vi "4ChNCS_BIOPAC_dyspnea.vi"() -> ()   [LabVIEW 2016]
uses:
  <instrlib>/niUSRP/niUSRP Timestamp.ctl
  <vilib>/Utility/miscctls.llb/LVDateTimeRec.ctl
  <vilib>/Analysis/3filter.llb/Filter Passband Type.ctl
  <vilib>/sound2/lvsound2.llb/Sampling Mode.ctl
  <instrlib>/niUSRP/niUSRP Configure Time Start Trigger.vi
  <vilib>/Platform/browser.llb/Open URL in Default Browser (string).vi
  <instrlib>/niUSRP/niUSRP Write Tx Data (2D CDB).vi
  <instrlib>/niUSRP/niUSRP Fetch Rx Data (2D CDB).vi
  <vilib>/Analysis/3filter.llb/Butterworth Filter (DBL).vi
  <vilib>/Analysis/3filter.llb/Butterworth Filter (CDB).vi
  <vilib>/sound2/lvsound2.llb/Sound File Info (path).vi
  <vilib>/sound2/lvsound2.llb/Sound File Read Open.vi
  <vilib>/sound2/lvsound2.llb/Sound File Read (DBL).vi
  <vilib>/sound2/lvsound2.llb/Sound Output Write (DBL).vi
  <vilib>/measure/NI_MABase.lvlib
  <vilib>/Analysis/NI_AALBase.lvlib
  Program Files (x86)/BIOPAC Systems, Inc/BIOPAC Hardware API 2.2 Education/x64/mpdev.dll
panel:
  in  "Mute":bool
  out "Play Sound":bool=TRUE
  in  "bottom filter":T1
  in  "top filter":T1=enum."Bandpass"
  out "Acq Started":bool
  out "# BIO View Q":i32
  out "# BIO Buffer":i32
  out "Boolean":bool=TRUE
  out "Disconnecting":bool
  out "Stopping":bool
  out "Connecting":bool
  out "Disconnected":bool
  in  "Show BIO":bool
  out "# BIOViewQ2":i32
  out "Array 1 View":dbl[](graph)
  out "Array 2 View":dbl[](graph)
  out "Array 3 View":dbl[](graph)
  out "Array 4 View":dbl[](graph)
  out "View Array Size":i32
  out "# Elements in Array":i32
  out "ACQ -# Elements":i32
  out "Receive Success":bool
  out "# ACQ cycles":i32
  out "Bytes Read":i32
  out "Bytes To Read":i32
  out "Receive Total Size":dbl format="%#_13g"
  out "Receiving":bool
  in  "Start Acquisition":bool
  in  "Disconnect":bool
  out "ACQ ms":dbl=250.0 format="%#_13g"
  in  "Stop Acquisition":bool
  out "Connected":bool
  in  "Sample Rate":dbl=1.0 caption="ms/sample" min=0.0
  in  "Analog Channels":i32[](array[numeric])=[1, 1, 1, 1]
  out "# Channels":dbl format="%#_13g"
  out "BIO Connect":i32
  in  "BIO Connect":bool=TRUE
  in  "OpenHTML":bool=TRUE
  in  "Abd (cm)":string="0"
  in  "Thorax (cm)":string="0"
  in  "Comments":string
  in  "Weight (lbs)":string="0"
  in  "Age (yrs)":string="0"
  in  "Sex":string(combo)="Female"
  in  "Height (cm)":string="0"
  in  "Case #":string="0"
  out "Start Time":T2
  out "Total Routine Time":dbl(slide) scale=0.0..300.0
  out "Elapsed Time":dbl caption="Elapsed Time (s)"
  out "Next Instruction":string
  out "Current Instruction":string
  in  "Routine Selection":T3(ring)
  out "Current Routine":string
  out "Tx3Rx4":dbl[](graph)
  out "Tx4Rx4":dbl[](graph)
  out "Tx4Rx3":dbl[](graph)
  out "Tx3Rx3":dbl[](graph)
  out "ChAmp":dbl[][](array[numeric])=[[1.7262327066457893e-05, 1.899698926539768e-05, 2.131979680782845e-05, 2.7507513862708948e-05, 3.236234947998919e-05, 3.384280863448985e-05, 3.3113712649913256e-05, 2.8744318806479064e-05, 2.4117959107532184e-05, 2.0714217164135817e-05, 1.7964639969242282e-05, 1.4127881869429752e-05, 1.5692535768228094e-05, 2.4152619914305532e-05, 2.8339686382715385e-05, 2.606906286720416e-05, 2.1755918570529384e-05, 2.0929028564145826e-05, 2.2419410493859248e-05, 2.1786896096171967e-05, 1.7145005999174206e-05, 1.5886785364638103e-05, 1.995380091360238e-05, 1.96084446445408e-05, 1.3881312052638574e-05, 5.368463432831762e-06, 7.886976522489036e-06, 1.718108126568357e-05, 1.984430714817916e-05, 1.8874058751572535e-05, 1.7869312672433515e-05, 1.7356735499504872e-05, 2.065235332503479e-05, 2.1951680154988656e-05, 2.0363547237431346e-05, 2.1229264430323524e-05, 2.188656276617781e-05, 2.1477411495382004e-05, 1.913194947952161e-05, 1.374906879007994e-05, 1.084407557924396e-05, 1.0538448835067238e-05, 1.3462486513328936e-05, 1.979383250422823e-05, 2.381539261154395e-05, 2.2167223174073578e-05, 1.7644503717147575e-05, 1.870536234643517e-05, 2.2751950524913166e-05, 2.340432192813861e-05, 2.2468849270761083e-05, 2.4188550691353842e-05, 2.7519058552290856e-05, 3.1102581077866726e-05, 3.580393911829494e-05, 3.78912649503874e-05, 3.327873597801261e-05, 2.4510981949940783e-05, 1.8465065354817837e-05, 1.7132224969133005e-05, 1.7642310138371268e-05, 1.88142956741822e-05, 1.560032046277488e-05, 9.753217862235494e-06, 1.2015090850038981e-05, 1.776834560720681e-05, 2.4803861691952522e-05, 2.8043624192078222e-05, 2.684382525540612e-05, 2.3530222840588965e-05, 2.0528849124310057e-05, 1.9668374613316667e-05, 1.9146637114645684e-05, 1.5474488036915515e-05, 1.739488550213199e-05, 2.5095299380068926e-05, 3.2858145215540916e-05, 3.439509649081835e-05, 2.6143868318774837e-05, 1.7977385637690134e-05, 1.6384181575586158e-05, 1.4888284293264162e-05, 1.1597491470576354e-05, 1.1445555578759772e-05, 1.4980688444081562e-05, 1.909173519498907e-05, 1.9461150455264684e-05, 1.845876729070065e-05, 1.8005010185132642e-05, 1.9028924898462435e-05, 1.7575955788217445e-05, 1.4184298105937452e-05, 9.414371560237339e-06, 5.4356042784590255e-06, 8.10928562517548e-06, 9.28876849225871e-06, 8.695785214389758e-06, 1.2695777397634576e-05, 1.6809431598631123e-05, 2.1908643727461497e-05], [0.39904903865563796, 0.39903176051530775, 0.39902405260596024, 0.3990221650023599, 0.3990182934858042, 0.39901299641778676, 0.39900459263010085, 0.39899398548309095, 0.3989851312683333, 0.3989817758172843, 0.39898441600096285, 0.3989920701551657, 0.3989957319087615, 0.3989970252526829, 0.3990014639144786, 0.3990082495650084, 0.39901677157837184, 0.39902202434845035, 0.3990170521098724, 0.3990061914814684, 0.39899957115083645, 0.39900163440594105, 0.39901134932465093, 0.3990245430143365, 0.3990299364956871, 0.3990206423396574, 0.39901294696264844, 0.399015237964853, 0.3990195320664335, 0.3990239908891069, 0.39902678858482366, 0.3990303142377581, 0.3990363654196349, 0.39903798034344395, 0.39903568308022536, 0.3990295778239386, 0.3990213145612541, 0.3990115641317417, 0.3990031911721688, 0.3990044335692754, 0.3990142055365442, 0.3990231880559529, 0.3990294810791408, 0.39903152543597487, 0.3990303417237137, 0.39902587131491124, 0.39902317862698444, 0.3990231908517323, 0.3990187535042287, 0.39901147460102687, 0.39900466569609977, 0.399000198693456, 0.398994572076958, 0.39898792975360287, 0.39898351183081265, 0.39898252129559103, 0.3989860199605185, 0.3989908704807006, 0.39899345184972185, 0.39899268675930705, 0.39898929894357515, 0.39898974479144206, 0.3989970434213525, 0.39900457970685, 0.3990084272376425, 0.3990059437407563, 0.39900092658003017, 0.3989998521554356, 0.3989999155043143, 0.39900335732390085, 0.3990086633280822, 0.39901161043288735, 0.3990153435576799, 0.3990232290578827, 0.39902895125044885, 0.3990233171970213, 0.39901091768095076, 0.3989963560226853, 0.3989823146041765, 0.39898013105698543, 0.39899131681473166, 0.3990088743561722, 0.39902163871137375, 0.39902552269435965, 0.3990216751013488, 0.3990108271690995, 0.3989999368161602, 0.39899179748001445, 0.3989869444795569, 0.3989823014007489, 0.3989811018380635, 0.3989866085692465, 0.3989974881575293, 0.399009653455826, 0.39902039237597164, 0.39903113834388676, 0.39903799466445666, 0.39903656085835637, 0.39902912933239515, 0.3990196685727854], [0.5089284260094796, 0.5089413529092005, 0.5089385924023097, 0.5089461735853302, 0.5089333321440155, 0.5089367652503622, 0.5089376331435306, 0.5089306671430541, 0.508949239645895, 0.5089486561361645, 0.5089529378833244, 0.5089419476875585, 0.5089298840108731, 0.5089475772042052, 0.5089441426339854, 0.5089427381450184, 0.5089483329108746, 0.5089280151098653, 0.5089336602793385, 0.5089062019851882, 0.5089074628030626, 0.5088932174425751, 0.5088701289561509, 0.5088760830698362, 0.5088683341509143, 0.5088818393635381, 0.5089000365985035, 0.5088962730652971, 0.5089053012825656, 0.5088919060061875, 0.5088858810710211, 0.5088778714303226, 0.508862396898039, 0.5088799706522465, 0.508890020250467, 0.5089068411749241, 0.508910151200762, 0.5088879724716624, 0.5088963605339264, 0.5088989546591678, 0.5089079531975655, 0.5089307483176185, 0.5089353690581762, 0.5089322510910641, 0.5089226818391756, 0.5089231205950179, 0.5089421889187917, 0.5089302121637822, 0.5089288553338916, 0.5089136387417116, 0.5088923938634197, 0.5088806790242092, 0.5088543127997475, 0.5088388632427274, 0.5088290815518671, 0.5088136498514574, 0.508828716232115, 0.5088373004254244, 0.5088536031198835, 0.5088663652543981, 0.5088663647379902, 0.5088663839922184, 0.5088589552438861, 0.5088642449634635, 0.5088725023266256, 0.5088718014416865, 0.5088674063260687, 0.5088515437004615, 0.5088682831786894, 0.5088713788197812, 0.5088809924897628, 0.508878513506942, 0.5088771181893693, 0.5088848435184512, 0.5088770842370816, 0.5088914766511436, 0.5089003523667647, 0.5089066301516674, 0.5089314320882471, 0.5089402101447223, 0.508962553406896, 0.5089753861787446, 0.5089593307295952, 0.5089478542324088, 0.5089278310589712, 0.5089248500720587, 0.5089163513653545, 0.5089005689237424, 0.5089083211616405, 0.5088993300683022, 0.5088927412237987, 0.5088830866377116, 0.5088718481995638, 0.5088897909905771, 0.5088809733102648, 0.5088790935282286, 0.5088680814653207, 0.5088523600270333, 0.5088613943195607, 0.5088543176402154], [2.0662941946213977e-05, 2.282608405319783e-05, 2.237600508813514e-05, 2.2542693256186783e-05, 2.041826329305299e-05, 1.6288400811782785e-05, 1.0891495139698275e-05, 1.4190599881567273e-05, 1.8742691366266016e-05, 1.8736119036749436e-05, 1.741774537028846e-05, 1.5658954058158222e-05, 1.5904856683822096e-05, 1.6871005066910787e-05, 1.5599249074465836e-05, 1.3520520470394872e-05, 1.3927163947888679e-05, 1.5334805249818678e-05, 1.4564830067379515e-05, 9.817520346860189e-06, 1.3098820613974226e-05, 1.929550220456421e-05, 2.3072255815616586e-05, 2.4321951176986116e-05, 2.3250917563816834e-05, 2.1644284217119052e-05, 1.7041306350033735e-05, 1.0688883027066213e-05, 9.28433634468159e-06, 1.1420718289762068e-05, 1.7056250213804775e-05, 1.9836991189555113e-05, 1.746716828521344e-05, 1.2441527630540996e-05, 8.566795426917848e-06, 9.815076354382859e-06, 1.0229272880058857e-05, 9.936691802926115e-06, 1.536494187514889e-05, 2.3346259934086635e-05, 2.7477587888222747e-05, 2.882421007601368e-05, 2.763067836551142e-05, 2.1577345489474273e-05, 1.3485424327083916e-05, 9.52579824483287e-06, 1.3113651673496717e-05, 1.5276095683726537e-05, 1.6308973250379756e-05, 1.8045078515596545e-05, 1.7849042225306495e-05, 1.2607829522468473e-05, 7.109107971268437e-06, 6.6038815895810515e-06, 6.924972052119899e-06, 4.965235247536195e-06, 5.757305113334596e-06, 9.21497446069365e-06, 9.781248515919794e-06, 1.0683021318304504e-05, 1.196938592791573e-05, 1.159802409297526e-05, 1.012272777630437e-05, 9.65935822948268e-06, 1.4116839432017005e-05, 1.847684147148342e-05, 1.6783927528588872e-05, 1.0863513026975652e-05, 7.650914818223192e-06, 9.456183557358687e-06, 1.0426180609097815e-05, 8.567604650724215e-06, 8.546559610017728e-06, 1.2946532793024891e-05, 1.7245567743458815e-05, 2.0097444147186203e-05, 2.0459407417437442e-05, 1.9957232554286306e-05, 1.996659645997603e-05, 1.7332136966233293e-05, 1.5115608112097958e-05, 1.762095864401886e-05, 1.992020410454883e-05, 2.0585166404108466e-05, 2.212056735942569e-05, 2.2957279986002272e-05, 2.3103396847026532e-05, 2.320807116373638e-05, 2.0818984342366494e-05, 1.789850158592137e-05, 1.64936985167028e-05, 1.4204813599995013e-05, 1.2878752736428332e-05, 1.4757379916553103e-05, 1.713867099725903e-05, 1.6105166890214558e-05, 1.20593443919334e-05, 1.2171370167939264e-05, 1.2336933066341984e-05, 1.1620987924410626e-05]]
  out "Output":bool=TRUE
  out "Ch4 Amplitude":dbl step=0.05 format="%#.6g"
  out "Ch3 Amplitude":dbl=0.25 step=0.05 format="%#.6g"
  out "Ch2 Amplitude":dbl=0.6 step=0.05 format="%#.6g"
  out "Ch1 Amplitude":dbl step=0.05 format="%#.6g"
  out "Tx1Rx2":dbl[](graph)
  out "Tx2Rx2":dbl[](graph)
  out "Tx2Rx1":dbl[](graph)
  out "Dis Sampling Rate":dbl=1000.0 format="%#_6p"
  in  "DownSamplingRatio 2":i32=10
  out "Sampling Rate":dbl=10000.0 format="%#_6p"
  out "Flush":bool
  out "8 Ch Heart":dbl[][](array[numeric])
  out "NCS Save Loops":i32=56132
  out "Save":bool
  out "# NCS Buffer":i32
  out "Buffer":bool
  in  "fl Bottom":dbl=10.0 format="%0.4f"
  in  "fh Bottom":dbl=20.0 format="%0.2f"
  in  "DownSamplingRatio1":i32=100
  in  "fl Top":dbl=4.0 format="%0.4f"
  in  "fh Top":dbl=20.0 format="%0.2f"
  out "# elements in view queue":i32
  out "Tx1Rx1":dbl[](graph)
  out "DownSamplingRatio":i32=100
  out "BW/2":dbl=1000.0
  out "# IQ queue Ch 2":i32
  out "# IQ queue Ch 1":i32
  in  "Dis2":bool=TRUE
  in  "Dis1":bool=TRUE
  out "IQ Graph 2":dbl[][](graph)
  out "IQ Graph":dbl[][](graph)
  out "Tx2 Waveform":cdb[][](array[numeric])
  out "Tx1 Waveform":cdb[][](array[numeric])
  in  "Ch3&4 carrier frequency [Hz] 2":dbl=1830000000.0 format="%#_6p"
  in  "Ch1&2 carrier frequency [Hz]":dbl=900000000.0 format="%#_6p"
  in  "Rx2 Gain 2":dbl=5.0 format="%#_6f"
  in  "Tx2 Gain 2":dbl=5.0 format="%#_6f"
  in  "Rx1 Gain 2":dbl=20.0 format="%#_6f"
  in  "Tx1 Gain 2":dbl=20.0 format="%#_6f"
  out "error out 2":errorcluster
  in  "Start Trigger Time 2":T4={"whole seconds"=1, "fractional seconds"=0.0}
  in  "Channel 4 Tone Amplitude":dbl=0.5 step=0.05 format="%#.6g"
  in  "Channel 4 Tone Frequency":dbl=430000.0 format="%#_6p"
  in  "Channel 3 Tone Amplitude":dbl=0.5 step=0.05 format="%#.6g"
  in  "Channel 3 Tone Frequency":dbl=473000.0 format="%#_6p"
  out "Tx2 Waveform Graph":waveform(dbl)[](graph)=[{"t0"=timestamp(0.45999999999999996 s since 1904-01-01), "dt"=1e-06, "Y"=array[10000 elements]}, {"t0"=timestamp(0.45999999999999996 s since 1904-01-01), "dt"=1e-06, "Y"=array[10000 elements]}, {"t0"=timestamp(0.45999999999999996 s since 1904-01-01), "dt"=1e-06, "Y"=array[10000 elements]}, {"t0"=timestamp(0.45999999999999996 s since 1904-01-01), "dt"=1e-06, "Y"=array[10000 elements]}]
  in  "Waveform Size 2":dbl=10000.0
  in  "Stop 2":bool
  in  "Device Name 2":refnum<k15>="MyB210_2"
  in  "Tx2 Gain 1":dbl=5.0 format="%#_6f"
  in  "Tx IQ Rate 2":dbl=1000000.0 format="%#_6p"
  in  "Rx2 Gain 1":dbl=5.0 format="%#_6f"
  in  "Rx IQ Rate 2":dbl=1000000.0 format="%#_6p"
  out "error out 1":errorcluster
  in  "Start Trigger Time":T4={"whole seconds"=1, "fractional seconds"=0.0}
  in  "Stop":bool
  in  "Channel 2 Tone Amplitude":dbl=0.5 step=0.05 format="%#.6g"
  in  "Channel 2 Tone Frequency":dbl=440000.0 format="%#_6p"
  in  "Channel 1 Tone Amplitude":dbl=0.5 step=0.05 format="%#.6g"
  in  "Channel 1 Tone Frequency":dbl=355000.0 format="%#_6p"
  out "Tx1 Waveform Graph":waveform(dbl)[](graph)=[{"t0"=timestamp(0.45999999999999996 s since 1904-01-01), "dt"=1e-06, "Y"=array[10000 elements]}, {"t0"=timestamp(0.45999999999999996 s since 1904-01-01), "dt"=1e-06, "Y"=array[10000 elements]}, {"t0"=timestamp(0.45999999999999996 s since 1904-01-01), "dt"=1e-06, "Y"=array[10000 elements]}, {"t0"=timestamp(0.45999999999999996 s since 1904-01-01), "dt"=1e-06, "Y"=array[10000 elements]}]
  in  "Waveform Size 1":dbl=10000.0
  in  "Device Name":refnum<k15>="MyB210_1"
  in  "Tx1 Gain 1":dbl=20.0 format="%#_6f"
  in  "Tx IQ Rate 1":dbl=1000000.0 format="%#_6p"
  in  "Rx1 Gain 1":dbl=20.0 format="%#_6f"
  in  "Rx IQ Rate 1":dbl=1000000.0 format="%#_6p"
  # "Misc"
  # "Tx Waveform"
  # "IQ waveform"
  # "NCS"
  # "Channel Settings"
  # "Channel 1"
  # "Device Settings"
  # "BIO"
  # "Channel 2"
  # "Filters"
  # "Buffers"
  # "BIOPAC Connection"
  # "Channel 3"
  # "Post Study Survey:"
  # "https://cornell.qualtrics.com/jfe/form/SV_9QryoqkUKquSXD7"
  # "Channel 4"
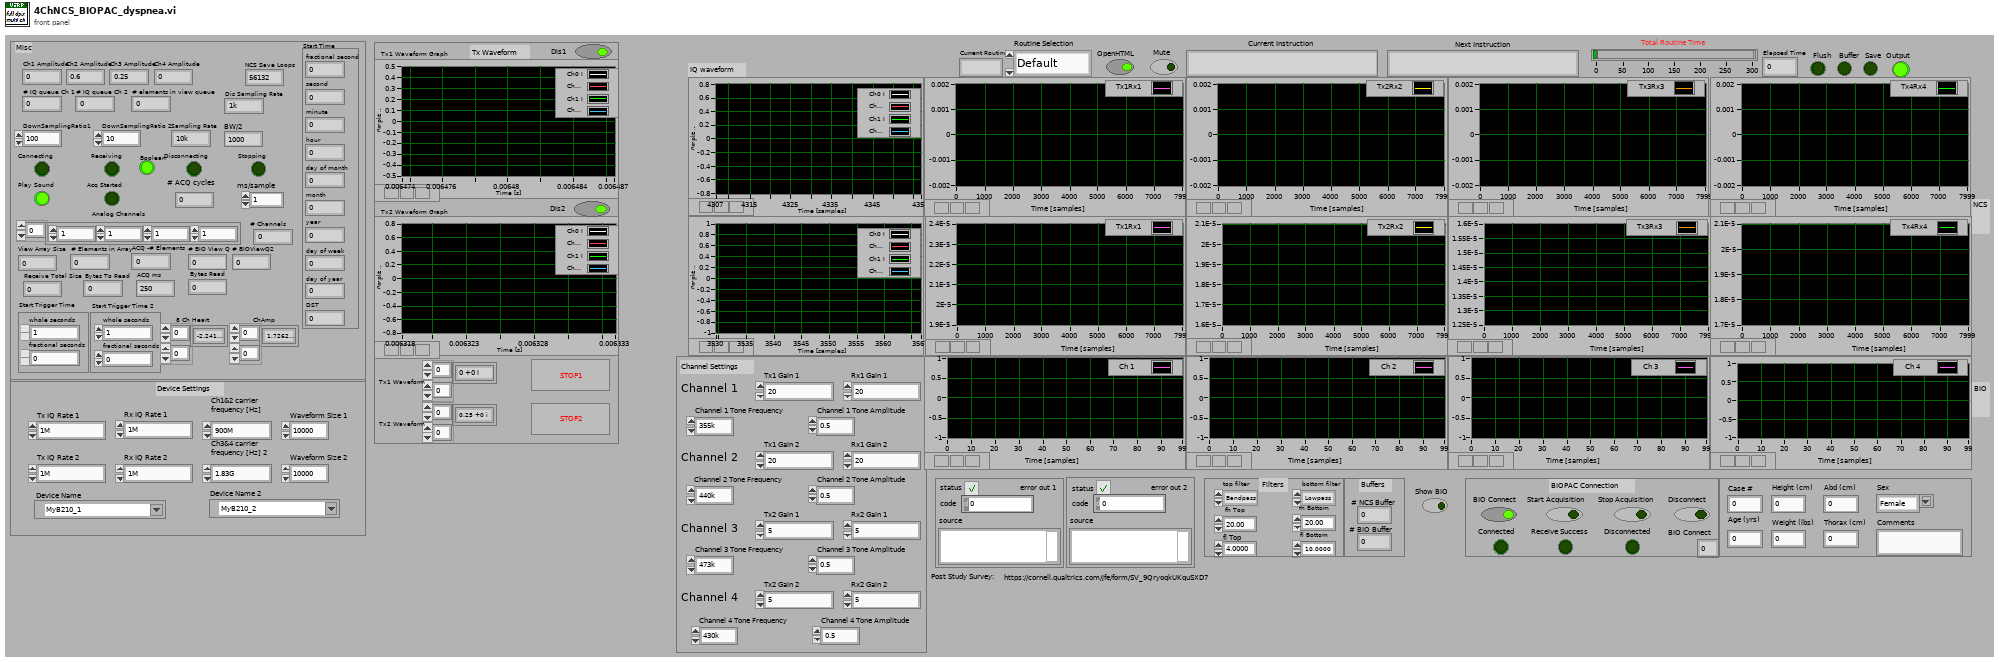
[diagram p1: front panel]
types:
  T1 = typedef "NI_AALBase.lvlib/Filter Passband Type.ctl" = enum32{"Lowpass", "Highpass", "Bandpass", "Bandstop"}
  T2 = typedef "LVDateTimeRec.ctl" = cluster{"fractional second":dbl, "second":i32, "minute":i32, "hour":i32, "day of month":i32, "month":i32, "year":i32, "day of week":i32, "day of year":i32, "DST":i32}
  T3 = enum16{"Default", "Test Run", "Training", "Routine 1", "Routine 2", "Routine 3", "Routine 4", "Routine 5a", "Routine 5b"}
  T4 = typedef "niUSRP Timestamp.ctl" = cluster{"whole seconds":u64, "fractional seconds":dbl}
  T5 = typedef "Sampling Mode.ctl" = i32
  T6 = typedef "Sound Data Format.ctl" = cluster{"sample rate (S/s)":dbl, "number of channels":i32, "bits per sample":i32}
  T7 = typedef "Sound File Refnum.ctl" = refnum<file>
  T8 = typedef "Sound Output Task ID.ctl" = u32
  T9 = enum16{"open", "open or create", "create or replace", "create", "open (read-only)"}
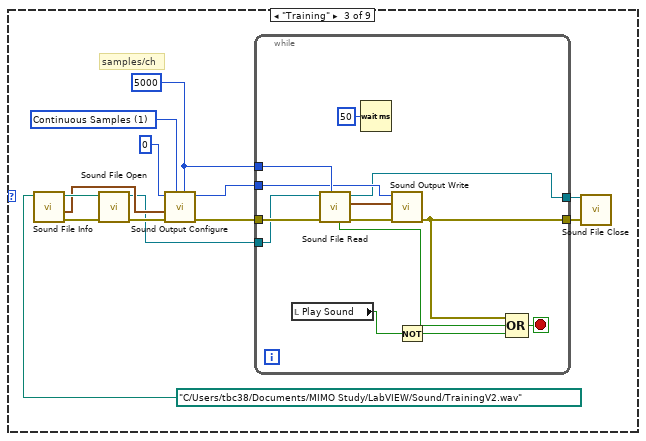
[diagram p5: hidden frame]
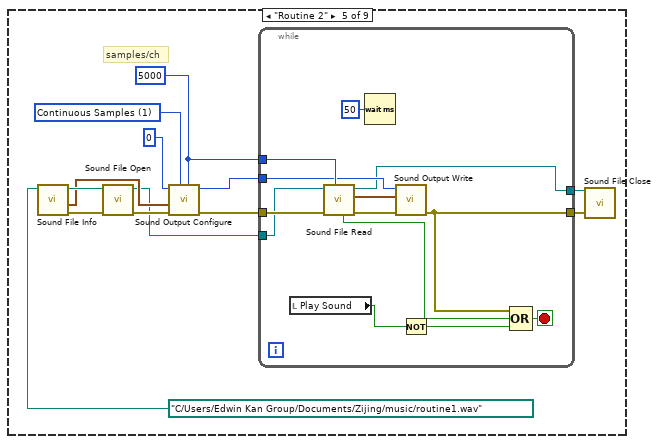
[diagram p7: hidden frame]
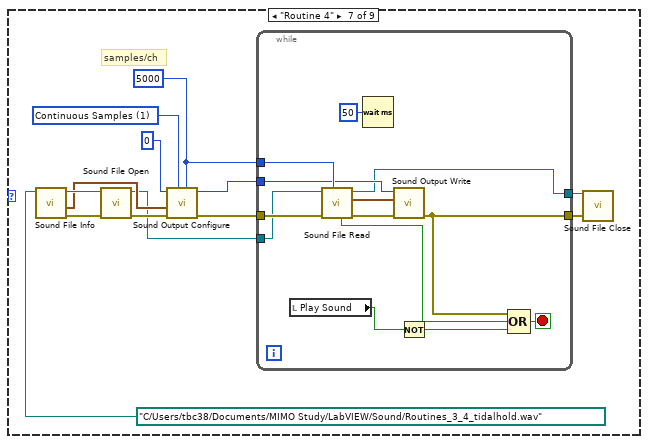
[diagram p8: hidden frame]
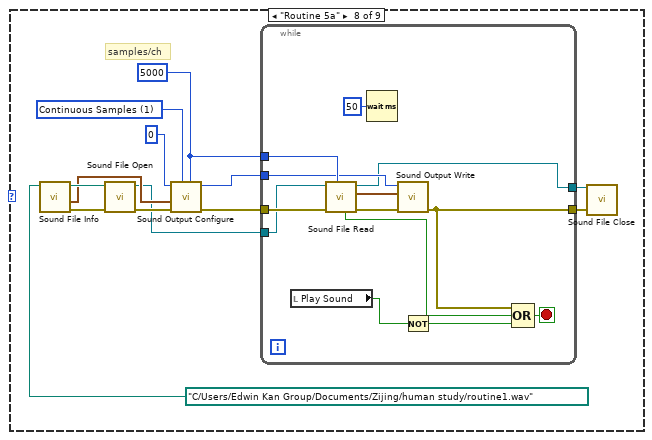
[diagram p9: hidden frame]
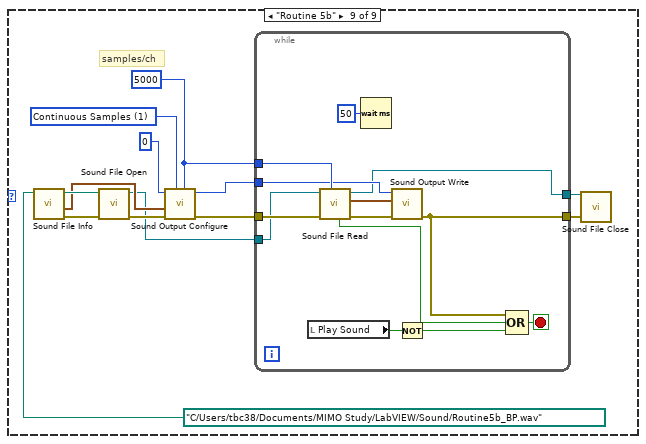
[diagram p10: hidden frame]
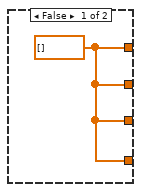
[diagram p11: hidden frame]
diagram:
  w1 = FALSE
  w29 = enum16{"Default"}."Default"
  w26 = 0.0 ("element")
  w27 = 800 ("dimension size")
  w33 = 4 ("dimension size")
  (unwired) 10
  w85 = "RX2"  # Tx active antenna
  w86 = "RX2"  # Tx active antenna
  w142 = 1 items=["Now", "Next Timebase Edge"] ("apply timestamp")
  w114 = "TX1"  # Tx active antenna
  w208 = 1 items=["Now", "Next Timebase Edge"] ("apply timestamp")
  w180 = "TX1"  # Tx active antenna
  # "Sound"
  # "Get it so that it acquires the proper number of cycles for the routine time. Front should be save synchronized"
  # "BIOPAC QUEUE"
  # "Current Sync Method:\nStart Buffering as soon as Acquisition Starts"
  # "Biopac Code. Use the flags to switch between these loops.\nCONNECT- Run to connect to the BIOPAC. Acquisition will not start. 'Connect Success' returns the status of this function.\nSTART ACQUISITION- Run to begin acquiring data from the BIOPAC. SYNCHRONIZATION IS IMPORTANT HERE.\nSTOP ACQUISITION- Run to stop acquiring data. The BIOPAC will disconnect and reconnect to prepare for another acquisition.\nDISCONNECT- Run to disconnect from BIOPAC. This will prohibit connection until the VI is restarted.\nSHOW/VIEWING- Dequeues the elements and displays them."
  # "Routine selection and implementation Loop"
  # "DownSamplingRatio"
  # "Set the attributes \nspecific to channel 1."
  # "Set the attributes \nspecific to channel 0."
  # "Set the attributes \nused by both Rx channels"
  # "Set the attributes \nspecific to Rx channel 1."
  # "Set the attributes \nspecific to Rx channel 0."
  # "Set the attributes \nspecific to channel 1."
  # "Set the attributes \nspecific to channel 0."
  # "Set the attributes \nused by both Rx channels"
  # "Set the attributes \nspecific to Rx channel 1."
  # "Set the attributes \nspecific to Rx channel 0."
  n1 = local write "BIO Connect"(w1) -> ()
  n2 = local write "Start Acquisition"(w1) -> ()
  n3 = local write "Stop Acquisition"(w1) -> ()
  n4 = local write "Disconnect"(w1) -> ()
  n5 = local write "Show BIO"(w1) -> ()
  n6 = local read "Device Name 2"() -> (w150:refnum<k15>)
  n7 = while {
    stop <- FALSE stop-if-true
    n8 = Wait (ms)(milliseconds to wait=50) -> ()  [unwired: 1 out]
    n9 = Not(x="Mute") -> (.not. x?=w224:bool)
    n10 = case shown="True" w224 {
      frame False {
      }
      frame True {
        n11 = local read "Routine Selection"() -> (w227:T3)
        n12 = case shown="\"Routine 3\"" w227 {
          frame "Default", Default {
          }
          frame "Test Run" {
          }
          frame "Training" {
            w231 = 5000
            w234 = T5 1 items=["Finite Samples", "Continuous Samples"] ("sample mode")
            # "samples/ch"
            n13 = call-poly <vilib>:"Sound File Info.vi"("path"=path "C:/Users/tbc38/Documents/MIMO Study/LabVIEW/Sound/TrainingV2.wav") -> ("error out"=w239:errorcluster, "sound format"=w235:T6, "path out"=w240:path)  [unwired: 7 in, 1 out]
            n14 = call-poly <vilib>:"Sound File Open.vi"("error in (no error)"=w239, "path"=w240) -> ("error out"=w238:errorcluster, "sound file refnum"=w230:T7)  [unwired: 8 in]
            n15 = call <vilib>:"Sound Output Configure.vi"("number of samples/ch"=w231, "sample mode"=w234, "error in (no error)"=w238, "sound format"=w235, "device ID"=u32 0) -> ("error out"=w233:errorcluster, "task ID"=w232:T8)  [unwired: 5 in]
            n16 = while {
              tunnel: w233 -> [w251]
              tunnel: w232 -> [w252]
              tunnel: w231 -> [w253]
              tunnel: w230 -> [w250]
              tunnel: [w244] -> w229
              tunnel: [w248] -> w228
              stop <- w242 stop-if-true
              n17 = local read "Play Sound"() -> (w241:bool)
              n18 = call-poly <vilib>:"Sound File Read.vi"("number of samples/ch (-1: all)"=w253, "error in (no error)"=w251, "sound file refnum"=w250) -> ("error out"=w247:errorcluster, "data"=w246:waveform(dbl)[], "sound file refnum out"=w248:T7, "end of file?"=w245:bool)  [unwired: 4 in, 1 out]
              n19 = Wait (ms)(milliseconds to wait=50) -> ()  [unwired: 1 out]
              n20 = call-poly <vilib>:"Sound Output Write.vi"("error in (no error)"=w247, "data"=w246, "task ID"=w252) -> ("error out"=w244:errorcluster)  [unwired: 7 in, 1 out]
              n21 = Not(x=w241) -> (.not. x?=w243:bool)
              n22 = Compound Arithmetic op=OR(w244, w245, w243) -> (w242:bool)
            }
            n23 = call <vilib>:"Sound File Close.vi"("error in (no error)"=w229, "sound file refnum"=w228) -> ()  [unwired: 9 in, 1 out]
          }
          frame "Routine 1" {
          }
          frame "Routine 2" {
            w257 = 5000
            w260 = T5 1 items=["Finite Samples", "Continuous Samples"] ("sample mode")
            # "samples/ch"
            n24 = call-poly <vilib>:"Sound File Info.vi"("path"=path "C:/Users/Edwin Kan Group/Documents/Zijing/music/routine1.wav") -> ("error out"=w265:errorcluster, "sound format"=w261:T6, "path out"=w266:path)  [unwired: 7 in, 1 out]
            n25 = call-poly <vilib>:"Sound File Open.vi"("error in (no error)"=w265, "path"=w266) -> ("error out"=w264:errorcluster, "sound file refnum"=w256:T7)  [unwired: 8 in]
            n26 = call <vilib>:"Sound Output Configure.vi"("number of samples/ch"=w257, "sample mode"=w260, "error in (no error)"=w264, "sound format"=w261, "device ID"=u32 0) -> ("error out"=w259:errorcluster, "task ID"=w258:T8)  [unwired: 5 in]
            n27 = while {
              tunnel: w259 -> [w277]
              tunnel: w258 -> [w278]
              tunnel: w257 -> [w279]
              tunnel: w256 -> [w276]
              tunnel: [w270] -> w255
              tunnel: [w274] -> w254
              stop <- w268 stop-if-true
              n28 = local read "Play Sound"() -> (w267:bool)
              n29 = call-poly <vilib>:"Sound File Read.vi"("number of samples/ch (-1: all)"=w279, "error in (no error)"=w277, "sound file refnum"=w276) -> ("error out"=w273:errorcluster, "data"=w272:waveform(dbl)[], "sound file refnum out"=w274:T7, "end of file?"=w271:bool)  [unwired: 4 in, 1 out]
              n30 = Wait (ms)(milliseconds to wait=50) -> ()  [unwired: 1 out]
              n31 = call-poly <vilib>:"Sound Output Write.vi"("error in (no error)"=w273, "data"=w272, "task ID"=w278) -> ("error out"=w270:errorcluster)  [unwired: 7 in, 1 out]
              n32 = Not(x=w267) -> (.not. x?=w269:bool)
              n33 = Compound Arithmetic op=OR(w270, w271, w269) -> (w268:bool)
            }
            n34 = call <vilib>:"Sound File Close.vi"("error in (no error)"=w255, "sound file refnum"=w254) -> ()  [unwired: 9 in, 1 out]
          }
          frame "Routine 3" {
          }
          frame "Routine 4" {
            w283 = 5000
            w286 = T5 1 items=["Finite Samples", "Continuous Samples"] ("sample mode")
            # "samples/ch"
            n35 = call-poly <vilib>:"Sound File Info.vi"("path"=path "C:/Users/tbc38/Documents/MIMO Study/LabVIEW/Sound/Routines_3_4_tidalhold.wav") -> ("error out"=w291:errorcluster, "sound format"=w287:T6, "path out"=w292:path)  [unwired: 7 in, 1 out]
            n36 = call-poly <vilib>:"Sound File Open.vi"("error in (no error)"=w291, "path"=w292) -> ("error out"=w290:errorcluster, "sound file refnum"=w282:T7)  [unwired: 8 in]
            n37 = call <vilib>:"Sound Output Configure.vi"("number of samples/ch"=w283, "sample mode"=w286, "error in (no error)"=w290, "sound format"=w287, "device ID"=u32 0) -> ("error out"=w285:errorcluster, "task ID"=w284:T8)  [unwired: 5 in]
            n38 = while {
              tunnel: w285 -> [w303]
              tunnel: w284 -> [w304]
              tunnel: w283 -> [w305]
              tunnel: w282 -> [w302]
              tunnel: [w296] -> w281
              tunnel: [w300] -> w280
              stop <- w294 stop-if-true
              n39 = local read "Play Sound"() -> (w293:bool)
              n40 = call-poly <vilib>:"Sound File Read.vi"("number of samples/ch (-1: all)"=w305, "error in (no error)"=w303, "sound file refnum"=w302) -> ("error out"=w299:errorcluster, "data"=w298:waveform(dbl)[], "sound file refnum out"=w300:T7, "end of file?"=w297:bool)  [unwired: 4 in, 1 out]
              n41 = Wait (ms)(milliseconds to wait=50) -> ()  [unwired: 1 out]
              n42 = call-poly <vilib>:"Sound Output Write.vi"("error in (no error)"=w299, "data"=w298, "task ID"=w304) -> ("error out"=w296:errorcluster)  [unwired: 7 in, 1 out]
              n43 = Not(x=w293) -> (.not. x?=w295:bool)
              n44 = Compound Arithmetic op=OR(w296, w297, w295) -> (w294:bool)
            }
            n45 = call <vilib>:"Sound File Close.vi"("error in (no error)"=w281, "sound file refnum"=w280) -> ()  [unwired: 9 in, 1 out]
          }
          frame "Routine 5a" {
            w309 = 5000
            w312 = T5 1 items=["Finite Samples", "Continuous Samples"] ("sample mode")
            # "samples/ch"
            n46 = call-poly <vilib>:"Sound File Info.vi"("path"=path "C:/Users/Edwin Kan Group/Documents/Zijing/human study/routine1.wav") -> ("error out"=w317:errorcluster, "sound format"=w313:T6, "path out"=w318:path)  [unwired: 7 in, 1 out]
            n47 = call-poly <vilib>:"Sound File Open.vi"("error in (no error)"=w317, "path"=w318) -> ("error out"=w316:errorcluster, "sound file refnum"=w308:T7)  [unwired: 8 in]
            n48 = call <vilib>:"Sound Output Configure.vi"("number of samples/ch"=w309, "sample mode"=w312, "error in (no error)"=w316, "sound format"=w313, "device ID"=u32 0) -> ("error out"=w311:errorcluster, "task ID"=w310:T8)  [unwired: 5 in]
            n49 = while {
              tunnel: w311 -> [w329]
              tunnel: w310 -> [w330]
              tunnel: w309 -> [w331]
              tunnel: w308 -> [w328]
              tunnel: [w322] -> w307
              tunnel: [w326] -> w306
              stop <- w320 stop-if-true
              n50 = local read "Play Sound"() -> (w319:bool)
              n51 = call-poly <vilib>:"Sound File Read.vi"("number of samples/ch (-1: all)"=w331, "error in (no error)"=w329, "sound file refnum"=w328) -> ("error out"=w325:errorcluster, "data"=w324:waveform(dbl)[], "sound file refnum out"=w326:T7, "end of file?"=w323:bool)  [unwired: 4 in, 1 out]
              n52 = Wait (ms)(milliseconds to wait=50) -> ()  [unwired: 1 out]
              n53 = call-poly <vilib>:"Sound Output Write.vi"("error in (no error)"=w325, "data"=w324, "task ID"=w330) -> ("error out"=w322:errorcluster)  [unwired: 7 in, 1 out]
              n54 = Not(x=w319) -> (.not. x?=w321:bool)
              n55 = Compound Arithmetic op=OR(w322, w323, w321) -> (w320:bool)
            }
            n56 = call <vilib>:"Sound File Close.vi"("error in (no error)"=w307, "sound file refnum"=w306) -> ()  [unwired: 9 in, 1 out]
          }
          frame "Routine 5b" {
            w335 = 5000
            w338 = T5 1 items=["Finite Samples", "Continuous Samples"] ("sample mode")
            # "samples/ch"
            n57 = call-poly <vilib>:"Sound File Info.vi"("path"=path "C:/Users/tbc38/Documents/MIMO Study/LabVIEW/Sound/Routine5b_BP.wav") -> ("error out"=w343:errorcluster, "sound format"=w339:T6, "path out"=w344:path)  [unwired: 7 in, 1 out]
            n58 = call-poly <vilib>:"Sound File Open.vi"("error in (no error)"=w343, "path"=w344) -> ("error out"=w342:errorcluster, "sound file refnum"=w334:T7)  [unwired: 8 in]
            n59 = call <vilib>:"Sound Output Configure.vi"("number of samples/ch"=w335, "sample mode"=w338, "error in (no error)"=w342, "sound format"=w339, "device ID"=u32 0) -> ("error out"=w337:errorcluster, "task ID"=w336:T8)  [unwired: 5 in]
            n60 = while {
              tunnel: w337 -> [w355]
              tunnel: w336 -> [w356]
              tunnel: w335 -> [w357]
              tunnel: w334 -> [w354]
              tunnel: [w348] -> w333
              tunnel: [w352] -> w332
              stop <- w346 stop-if-true
              n61 = local read "Play Sound"() -> (w345:bool)
              n62 = call-poly <vilib>:"Sound File Read.vi"("number of samples/ch (-1: all)"=w357, "error in (no error)"=w355, "sound file refnum"=w354) -> ("error out"=w351:errorcluster, "data"=w350:waveform(dbl)[], "sound file refnum out"=w352:T7, "end of file?"=w349:bool)  [unwired: 4 in, 1 out]
              n63 = Wait (ms)(milliseconds to wait=50) -> ()  [unwired: 1 out]
              n64 = call-poly <vilib>:"Sound Output Write.vi"("error in (no error)"=w351, "data"=w350, "task ID"=w356) -> ("error out"=w348:errorcluster)  [unwired: 7 in, 1 out]
              n65 = Not(x=w345) -> (.not. x?=w347:bool)
              n66 = Compound Arithmetic op=OR(w348, w349, w347) -> (w346:bool)
            }
            n67 = call <vilib>:"Sound File Close.vi"("error in (no error)"=w333, "sound file refnum"=w332) -> ()  [unwired: 9 in, 1 out]
          }
        }
      }
    }
  }
  n68 = while {
    stop <- FALSE stop-if-true
    # "STOP ACQUISITION"
    n69 = local read "Connected"() -> (w362:bool)
    n70 = local read "Receiving"() -> (w361:bool)
    n71 = local read "Stopping"() -> (w359:bool)
    n72 = Wait (ms)(milliseconds to wait=100) -> ()  [unwired: 1 out]
    n73 = Not(x=w359) -> (.not. x?=w358:bool)
    n74 = And(x=w361, y=w358) -> (x .and. y?=w360:bool)
    n75 = And(x=w362, y=w360) -> (x .and. y?=w363:bool)
    n76 = And(x="Stop Acquisition", y=w363) -> (x .and. y?=w366:bool)
    n77 = case shown="True" w366 {
      frame False {
      }
      frame True {
        n78 = flat-sequence {
          frame #0 {
            n79 = local write "Stopping"(TRUE) -> ()
            n80 = dll-call lib="C:/Program Files (x86)/BIOPAC Systems, Inc/BIOPAC Hardware API 2.2 Education/x64/mpdev.dll" fn="stopAcquisition" label="stop"() -> ()  [unwired: 4 in, 2 out]
            n81 = local write "Receiving"(FALSE) -> ()
          }
          frame #1 {
            n82 = dll-call lib="C:/Program Files (x86)/BIOPAC Systems, Inc/BIOPAC Hardware API 2.2 Education/x64/mpdev.dll" fn="disconnectMPDev" label="disconnect"() -> ()  [unwired: 4 in, 2 out]
          }
          frame #2 {
            n83 = local read "ACQ ms"() -> (w371:dbl)
            n84 = Add(x=w371, y=200) -> (x+y=w372:dbl)
            n85 = Wait (ms)(milliseconds to wait=w372) -> ()  [unwired: 1 out]
          }
          frame #3 {
            w373 = FALSE
            n86 = local write "Stop Acquisition"(w373) -> ()
            n87 = local write "Stopping"(w373) -> ()
            n88 = local write "Connected"(w373) -> ()
            n89 = local write "Receive Success"(w373) -> ()
          }
        }
      }
    }
  }
  n90 = while {
    stop <- FALSE stop-if-true
    # "CONNECT"
    n91 = local read "Connecting"() -> (w382:bool)
    n92 = local read "Connected"() -> (w381:bool)
    n93 = local read "Disconnected"() -> (w378:bool)
    n94 = Wait (ms)(milliseconds to wait=500) -> ()  [unwired: 1 out]
    n95 = Not(x=w382) -> (.not. x?=w380:bool)
    n96 = Not(x=w381) -> (.not. x?=w377:bool)
    n97 = Not(x=w378) -> (.not. x?=w376:bool)
    n98 = And(x=w377, y=w376) -> (x .and. y?=w375:bool)
    n99 = And(x=w380, y=w375) -> (x .and. y?=w379:bool)
    n100 = And(x="BIO Connect", y=w379) -> (x .and. y?=w383:bool)
    n101 = case shown="True" w383 {
      frame False {
      }
      frame True {
        n102 = flat-sequence {
          frame #0 {
            n103 = local write "BIO Connect"(FALSE) -> ()
            n104 = local write "Connecting"(TRUE) -> ()
          }
          frame #1 {
            w393 = u32 1  # MPSUCCESS
            w402 = 10  # Enumeration Value For USB
            w401 = 103  # Enumeration Value for MP36
            n105 = String To Byte Array(string="") -> (unsigned byte array=w399:u8[])
            n106 = dll-call lib="C:/Program Files (x86)/BIOPAC Systems, Inc/BIOPAC Hardware API 2.2 Education/x64/mpdev.dll" fn="connectMPDev" label="connect"("mptype"=w401, "mpcomtype"=w402, "sn"=w399) -> ("return type"=w398:u32)  [unwired: 6 in, 2 out]
            "BIO Connect" <- w398
            n107 = Not Equal?(x=w398, y=w393) -> (x != y?=w397:bool)
            n108 = case shown="True" w397 {
              frame False {
              }
              frame True {
                n109 = flat-sequence {
                  frame #0 {
                    n110 = dll-call lib="C:/Program Files (x86)/BIOPAC Systems, Inc/BIOPAC Hardware API 2.2 Education/x64/mpdev.dll" fn="stopAcquisition" label="stop"() -> ()  [unwired: 4 in, 2 out]
                  }
                  frame #1 {
                    n111 = dll-call lib="C:/Program Files (x86)/BIOPAC Systems, Inc/BIOPAC Hardware API 2.2 Education/x64/mpdev.dll" fn="disconnectMPDev" label="disconnect"() -> ()  [unwired: 4 in, 2 out]
                  }
                }
              }
            }
            n112 = Not(x=w397) -> (.not. x?=w396:bool)
            n113 = case shown="True" w396 {
              tunnel: [w403 w405] -> w394
              tunnel: [w403 w404] -> w395
              frame False {
                w403 = 0
              }
              frame True {
                n114 = flat-sequence {
                  tunnel: [w409] -> w405
                  tunnel: [w411] -> w404
                  frame #0 {
                    n115 = To Double Precision Float(number="Analog Channels") -> (double precision float=w407:dbl[])
                    n116 = Add Array Elements(numeric array=w407) -> (sum=→"# Channels":dbl)
                    n117 = dll-call lib="C:/Program Files (x86)/BIOPAC Systems, Inc/BIOPAC Hardware API 2.2 Education/x64/mpdev.dll" fn="setAcqChannels" label="set analog CH"("aCH"="Analog Channels") -> ("return type"=w409:u32)  [unwired: 4 in, 2 out]
                  }
                  frame #1 {
                    n118 = dll-call lib="C:/Program Files (x86)/BIOPAC Systems, Inc/BIOPAC Hardware API 2.2 Education/x64/mpdev.dll" fn="setSampleRate" label="set sample rate"("rate"="Sample Rate") -> ("return type"=w411:u32)  [unwired: 4 in, 2 out]
                  }
                }
              }
            }
            n119 = Not Equal?(x=w395, y=w393) -> (x != y?=w390:bool)
            n120 = Not Equal?(x=w394, y=w393) -> (x != y?=w389:bool)
            n121 = Not(x=w389) -> (.not. x?=w391:bool)
            n122 = case shown="True" w389 {
              frame False {
              }
              frame True {
                n123 = flat-sequence {
                  frame #0 {
                    n124 = dll-call lib="C:/Program Files (x86)/BIOPAC Systems, Inc/BIOPAC Hardware API 2.2 Education/x64/mpdev.dll" fn="stopAcquisition" label="stop"() -> ()  [unwired: 4 in, 2 out]
                  }
                  frame #1 {
                    n125 = dll-call lib="C:/Program Files (x86)/BIOPAC Systems, Inc/BIOPAC Hardware API 2.2 Education/x64/mpdev.dll" fn="disconnectMPDev" label="disconnect"() -> ()  [unwired: 4 in, 2 out]
                  }
                }
              }
            }
            n126 = case shown="True" w390 {
              frame False {
              }
              frame True {
                n127 = flat-sequence {
                  frame #0 {
                    n128 = dll-call lib="C:/Program Files (x86)/BIOPAC Systems, Inc/BIOPAC Hardware API 2.2 Education/x64/mpdev.dll" fn="stopAcquisition" label="stop"() -> ()  [unwired: 4 in, 2 out]
                  }
                  frame #1 {
                    n129 = dll-call lib="C:/Program Files (x86)/BIOPAC Systems, Inc/BIOPAC Hardware API 2.2 Education/x64/mpdev.dll" fn="disconnectMPDev" label="disconnect"() -> ()  [unwired: 4 in, 2 out]
                  }
                }
              }
            }
            n130 = Not(x=w390) -> (.not. x?=w392:bool)
            n131 = And(x=w392, y=w391) -> (x .and. y?=w388:bool)
            n132 = local write "Connected"(w388) -> ()
          }
          frame #2 {
            n133 = local write "Connecting"(FALSE) -> ()
          }
        }
      }
    }
  }
  n134 = local read "Device Name"() -> (w216:refnum<k15>)
  n135 = call <instrlib>:"niUSRP Open Rx Session.vi"("device names"="Device Name 2") -> ("session handle out"=w141:refnum<k15>, "error out"=w140:errorcluster)  [unwired: 13 in]
  n136 = property class="niUSRP"(reference=w141, error in=w140, "Enabled Channels"="0,1" ("Configuration:Enabled Channels")) -> (reference out=w139:refnum<k15>, error out=w138:errorcluster)
  n137 = call <instrlib>:"niUSRP Open Rx Session.vi"("device names"="Device Name") -> ("session handle out"=w207:refnum<k15>, "error out"=w206:errorcluster)  [unwired: 13 in]
  n138 = property class="niUSRP"(reference=w207, error in=w206, "Enabled Channels"="0,1" ("Configuration:Enabled Channels")) -> (reference out=w205:refnum<k15>, error out=w204:errorcluster)
  n139 = call-poly <instrlib>:"niUSRP Configure Trigger.vi"("session handle"=w139, "start trigger time"="Start Trigger Time 2", "error in (no error)"=w138) -> ("session handle out"=w135:refnum<k15>, "error out"=w134:errorcluster)  [unwired: 11 in]
  n140 = call-poly <instrlib>:"niUSRP Configure Trigger.vi"("session handle"=w205, "start trigger time"="Start Trigger Time", "error in (no error)"=w204) -> ("session handle out"=w201:refnum<k15>, "error out"=w200:errorcluster)  [unwired: 11 in]
  n141 = property class="niUSRP"(reference=w135, error in=w134, "IQ Rate"="Rx IQ Rate 2") -> (reference out=w131:refnum<k15>, error out=w132:errorcluster)
  n142 = property class="niUSRP"(reference=w201, error in=w200, "IQ Rate"="Rx IQ Rate 1") -> (reference out=w197:refnum<k15>, error out=w198:errorcluster)
  n143 = property class="niUSRP" props=["Model", "Reference Frequency Source", "Timebase Clock Source"](reference=w197, error in=w198, "Reference Frequency Source"="RefIn" ("Clocking and Synchronization:Reference Frequency Source"), "Timebase Clock Source"="PpsIn" ("Clocking and Synchronization:Timebase Clock Source")) -> (reference out=w193:refnum<k15>, error out=w194:errorcluster)  [unwired: 1 out]
  n144 = property class="niUSRP" props=["Model", "Reference Frequency Source", "Timebase Clock Source"](reference=w131, error in=w132, "Reference Frequency Source"="RefIn" ("Clocking and Synchronization:Reference Frequency Source"), "Timebase Clock Source"="PpsIn" ("Clocking and Synchronization:Timebase Clock Source")) -> (reference out=w127:refnum<k15>, error out=w128:errorcluster)  [unwired: 1 out]
  n145 = local write "Routine Selection"(w29) -> ()
  n146 = local read "# Channels"() -> (w4:dbl)
  n147 = local read "ACQ ms"() -> (w3:dbl)
  n148 = while {
    shift-right: ["Routine Selection"] -> _
    shift-left: w29 -> [w419]
    stop <- FALSE stop-if-true
    n149 = case shown="\"Routine 3\"" w419 {
      tunnel: ["Default" w449 "Isovolumetric Training" "Routine1" "Routine2" "Routine3" "Routine4" "Routine5a" "Routine5b"] -> w420
      tunnel: [w434 w449 w458 w504 w552 w599 w632 w670 w696] -> w417
      tunnel: [w435 _ _ _ _ _ _ _ _] -> _
      tunnel: [w435 _ w456 w503 w546 w597 w627 w665 w691] -> w415
      tunnel: [w435 _ w456 w503 w546 w597 w627 w665 w691] -> w416
      tunnel: [w434 w449 w457 w502 w550 w600 w633 w671 w698] -> w414
      tunnel: [w433 w448 w455 w500 w549 w595 w636 w672 w693] -> w413
      frame "Default" {
        w435 = 0.0
        w434 = "No instruction"
        # "BIO should not be acquiring"
        # "If BIO is not connected, attempt to reconnect"
        n150 = Seconds To Date/Time(time stamp (now)=0.0) -> (date time rec=w433:T2)  [unwired: 1 in]
        n151 = local read "# NCS Buffer"() -> (w423:i32)
        n152 = Not Equal?(x=w423, y=0) -> (x != y?=w424:bool)
        n153 = local write "BIO Connect"(TRUE) -> ()
        n154 = case shown="True" w424 {
          frame False {
            n155 = local write "Flush"(FALSE) -> ()
          }
          frame True {
            "Flush" <- TRUE
          }
        }
        n156 = local write "Start Acquisition"(FALSE) -> ()
        n157 = local write "Stop Acquisition"(TRUE) -> ()
        "Save" <- FALSE
        "Buffer" <- FALSE
        "Output" <- FALSE
        "Play Sound" <- FALSE
      }
      frame "Test Run" {
        w449 = "Testing"
        # "Start BIO Acquisition"
        n158 = Seconds To Date/Time(time stamp (now)=0.0) -> (date time rec=w448:T2)  [unwired: 1 in]
        n159 = local write "Start Acquisition"(TRUE) -> ()
        n160 = local write "Stop Acquisition"(FALSE) -> ()
        n161 = local write "Play Sound"(FALSE) -> ()
        n162 = local write "Save"(FALSE) -> ()
        n163 = local write "Output"(TRUE) -> ()
        n164 = local write "Flush"(FALSE) -> ()
        n165 = local write "BIO Connect"(FALSE) -> ()
        n166 = local write "Buffer"(FALSE) -> ()
      }
      frame "Training" {
        w453 = 90.0  # Routine Time
        n167 = local read "Output"() -> (w450:bool)
        n168 = Not(x=w450) -> (.not. x?=w451:bool)
        n169 = call "Elapsed Time3"("Time Target (s)"=w453, "Reset"=w451) -> ("Get Start Time (s)"=w454:dbl, "Elapsed Time (s)"=w456:dbl, "Time has Elapsed"=w452:bool)  [unwired: 10 in, 5 out]
        n170 = script code="t = [300, ...\n       310, 313, 316, 319, 322, ...\n       340, 343, 346, 349, 352, ...\n       370, 373, 376, 379, 382, 390]; % 4) Isovol\nt = t-300;\n\nevent =  [0, ...\n                6, 3, 4, 5, 0, ... % 4) Isovol\n                7, 3, 4, 5, 0, ...\n                8, 3, 4, 5, 0, 0]; \n\nfor i = 2:length(t)\n    if ((x>=t(i-1)) &&  (x<t(i)))\n        y = event(i-1);\n        yNext = event(i);\n        % dt = t(i) - t(i-1);\n        break;\n    end\nend" "Routine timing"("x"=w456) -> ("yNext"=w459:dbl, "y"=w460:dbl)  [unwired: 1 in, 1 out]
        n171 = property on="Total Routine Time" class="Slide (strict)"("Scale.Maximum"=w453) -> ()  [unwired: 2 in, 2 out]
        n172 = Seconds To Date/Time(time stamp (now)=w454) -> (date time rec=w455:T2)  [unwired: 1 in]
        n173 = case shown="False" w452 {
          frame False {
            n174 = local write "Play Sound"(TRUE) -> ()
            n175 = local write "Output"(TRUE) -> ()
            n176 = local write "Flush"(FALSE) -> ()
            n177 = local write "Save"(FALSE) -> ()
            n178 = local write "Buffer"(FALSE) -> ()
            n179 = local write "Start Acquisition"(TRUE) -> ()
            n180 = local write "Stop Acquisition"(FALSE) -> ()
            n181 = local write "BIO Connect"(FALSE) -> ()
          }
          frame True {
            n182 = local write "Play Sound"(FALSE) -> ()
            n183 = local write "Buffer"(FALSE) -> ()
            n184 = local write "Output"(FALSE) -> ()
            n185 = local write "Save"(FALSE) -> ()
            n186 = local write "Flush"(FALSE) -> ()
            n187 = local write "Start Acquisition"(FALSE) -> ()
            n188 = local write "Stop Acquisition"(TRUE) -> ()
            n189 = local write "BIO Connect"(FALSE) -> ()
            n190 = local write "Routine Selection"(enum16{"Default"}."Default") -> ()
          }
        }
        n191 = case "Next Instruction" shown="3" w459 {
          tunnel: ["Perform Normal Breathing" "Max Inhale Breath Hold" "Max Exhalation Breath Hold" "Plug Nose. Move air to chest" "Allow abdomen to relax." "Move air to abdomen." "Exhale Fully" "Inhale Fully" "Inhale Partially"] -> w458
          frame 0, Default {
          }
          frame 1 {
          }
          frame 2 {
          }
          frame 3 {
          }
          frame 4 {
          }
          frame 5 {
          }
          frame 6 {
          }
          frame 7 {
          }
          frame 8 {
          }
        }
        n192 = case "Current Instruction" shown="5" w460 {
          tunnel: ["Perform Normal Breathing" "Max Inhale Breath Hold" "Max Exhalation Breath Hold" "Plug Nose. Move air to chest" "Allow abdomen to relax." "Move air to abdomen." "Exhale Fully" "Inhale Fully" "Inhale Partially"] -> w457
          frame 0, Default {
          }
          frame 1 {
          }
          frame 2 {
          }
          frame 3 {
          }
          frame 4 {
          }
          frame 5 {
          }
          frame 6 {
          }
          frame 7 {
          }
          frame 8 {
          }
        }
      }
      frame "Routine 1" {
        w507 = 300.0  # Routine Time
        # "390"
        # "Supine Breath Monitoring"
        n193 = local read "Output"() -> (w497:bool)
        n194 = Not(x=w497) -> (.not. x?=w498:bool)
        n195 = call "Elapsed Time"("Time Target (s)"=w507, "Reset"=w498) -> ("Get Start Time (s)"=w501:dbl, "Elapsed Time (s)"=w503:dbl, "Time has Elapsed"=w499:bool)  [unwired: 10 in, 5 out]
        n196 = script code="t = [0, 180, ...              % 1) Free breathing 3 mins\n       190, 200, 220, ...  % 2) Max inhale breath hold\n       250, 260, 280, ...  % 3) Max exhale breath hold\n       310, 313, 316, 319, 322, ...\n       340, 343, 346, 349, 352, ...\n       370, 373, 376, 379, 382, 390]; % 4) Isovol\n\nevent =  [0, 0, ...    % 1) Free breathing 3 mins\n                0, 1, 0, ... % 2) Max inhale breath hold\n                0, 2, 0, ... % 3) Max exhale breath hold\n                6, 3, 4, 5, 0, ... % 4) Isovol\n                7, 3, 4, 5, 0, ...\n                8, 3, 4, 5, 0, 0]; \n\nfor i = 2:length(t)\n    if ((x>=t(i-1)) &&  (x<t(i)))\n        y = event(i-1);\n        yNext = event(i);\n       % dt = t(i) - t(i-1);\n        break;\n    end\nend" "Routine timing"("x"=w503) -> ("yNext"=w505:dbl, "y"=w506:dbl)  [unwired: 1 in, 1 out]
        n197 = property on="Total Routine Time" class="Slide (strict)"("Scale.Maximum"=w507) -> ()  [unwired: 2 in, 2 out]
        n198 = Seconds To Date/Time(time stamp (now)=w501) -> (date time rec=w500:T2)  [unwired: 1 in]
        n199 = case shown="True" w499 {
          frame False {
            # "Routine Not Done. Continue buffering."
            n200 = flat-sequence {
              frame #0 {
                n201 = local write "Start Acquisition"(TRUE) -> ()
                n202 = local write "Stop Acquisition"(FALSE) -> ()
                n203 = local write "Output"(TRUE) -> ()
                n204 = local write "BIO Connect"(FALSE) -> ()
                n205 = local write "Play Sound"(TRUE) -> ()
              }
              frame #1 {
                n206 = local write "Buffer"(TRUE) -> ()
              }
            }
          }
          frame True {
            # "Routine done. Save."
            n207 = flat-sequence {
              frame #0 {
                n208 = local write "Buffer"(FALSE) -> ()
              }
              frame #1 {
                n209 = local write "Start Acquisition"(FALSE) -> ()
                n210 = local write "Stop Acquisition"(TRUE) -> ()
                n211 = local write "Output"(FALSE) -> ()
              }
              frame #2 {
                n212 = local write "Save"(TRUE) -> ()
              }
              frame #3 {
                n213 = Wait (ms)(milliseconds to wait=500) -> ()  [unwired: 1 out]
              }
              frame #4 {
                n214 = local write "Flush"(TRUE) -> ()
              }
              frame #5 {
                n215 = local write "Flush"(FALSE) -> ()
                n216 = local write "Save"(FALSE) -> ()
              }
              frame #6 {
                n217 = local write "Routine Selection"(enum16{"Default"}."Default") -> ()
                n218 = local write "Play Sound"(FALSE) -> ()
              }
            }
          }
        }
        n219 = case "Current Instruction" shown="6" w506 {
          tunnel: ["Perform Normal Breathing" "Max Inhale Breath Hold" "Max Exhalation Breath Hold" "Plug Nose. Move air to chest" "Allow abdomen to relax." "Move air to abdomen." "Exhale Fully" "Inhale Fully" "Inhale Partially"] -> w502
          frame 0, Default {
          }
          frame 1 {
          }
          frame 2 {
          }
          frame 3 {
          }
          frame 4 {
          }
          frame 5 {
          }
          frame 6 {
          }
          frame 7 {
          }
          frame 8 {
          }
        }
        n220 = case "Next Instruction" shown="3" w505 {
          tunnel: ["Perform Normal Breathing" "Max Inhale Breath Hold" "Max Exhalation Breath Hold" "Plug Nose. Move air to chest" "Allow abdomen to relax." "Move air to abdomen." "Exhale Fully" "Inhale Fully" "Inhale Partially"] -> w504
          frame 0, Default {
          }
          frame 1 {
          }
          frame 2 {
          }
          frame 3 {
          }
          frame 4 {
          }
          frame 5 {
          }
          frame 6 {
          }
          frame 7 {
          }
          frame 8 {
          }
        }
      }
      frame "Routine 2" {
        w554 = 180.0  # Routine Time
        # "Seated Breath Monitoring"
        n221 = local read "Output"() -> (w545:bool)
        n222 = Not(x=w545) -> (.not. x?=w544:bool)
        n223 = call "Elapsed Time2"("Time Target (s)"=w554, "Reset"=w544) -> ("Get Start Time (s)"=w548:dbl, "Elapsed Time (s)"=w546:dbl, "Time has Elapsed"=w547:bool)  [unwired: 10 in, 5 out]
        n224 = script code="t = [0, 180, ...              % 1) Free breathing 3 mins\n       190, 200, 220, ...  % 2) Max inhale breath hold\n       250, 260, 280, ...  % 3) Max exhale breath hold\n       310, 313, 316, 319, 322, ...\n       340, 343, 346, 349, 352, ...\n       370, 373, 376, 379, 382, 390]; % 4) Isovol\n\nevent =  [0, 0, ...    % 1) Free breathing 3 mins\n                0, 1, 0, ... % 2) Max inhale breath hold\n                0, 2, 0, ... % 3) Max exhale breath hold\n                6, 3, 4, 5, 0, ... % 4) Isovol\n                7, 3, 4, 5, 0, ...\n                8, 3, 4, 5, 0, 0]; \n\nfor i = 2:length(t)\n    if ((x>=t(i-1)) &&  (x<t(i)))\n        y = event(i-1);\n        yNext = event(i);\n       % dt = t(i) - t(i-1);\n        break;\n    end\nend" "Routine timing"("x"=w546) -> ("yNext"=w551:dbl, "y"=w553:dbl)  [unwired: 1 in, 1 out]
        n225 = property on="Total Routine Time" class="Slide (strict)"("Scale.Maximum"=w554) -> ()  [unwired: 2 in, 2 out]
        n226 = Seconds To Date/Time(time stamp (now)=w548) -> (date time rec=w549:T2)  [unwired: 1 in]
        n227 = case shown="True" w547 {
          frame False {
            # "Routine Not Done. Continue buffering."
            n228 = flat-sequence {
              frame #0 {
                n229 = local write "Play Sound"(TRUE) -> ()
                n230 = local write "Start Acquisition"(TRUE) -> ()
                n231 = local write "Output"(TRUE) -> ()
                n232 = local write "Stop Acquisition"(FALSE) -> ()
                n233 = local write "BIO Connect"(FALSE) -> ()
              }
              frame #1 {
                n234 = local write "Buffer"(TRUE) -> ()
              }
            }
          }
          frame True {
            # "Routine done. Save."
            n235 = flat-sequence {
              frame #0 {
                n236 = local write "Buffer"(FALSE) -> ()
              }
              frame #1 {
                n237 = local write "Output"(FALSE) -> ()
                n238 = local write "Start Acquisition"(FALSE) -> ()
                n239 = local write "Stop Acquisition"(TRUE) -> ()
              }
              frame #2 {
                n240 = local write "Save"(TRUE) -> ()
              }
              frame #3 {
                n241 = Wait (ms)(milliseconds to wait=500) -> ()  [unwired: 1 out]
              }
              frame #4 {
                n242 = local write "Flush"(TRUE) -> ()
              }
              frame #5 {
                n243 = local write "Flush"(FALSE) -> ()
                n244 = local write "Save"(FALSE) -> ()
              }
              frame #6 {
                n245 = local write "Routine Selection"(enum16{"Default"}."Default") -> ()
                n246 = local write "Play Sound"(FALSE) -> ()
              }
            }
          }
        }
        n247 = case "Current Instruction" shown="1" w553 {
          tunnel: ["Perform Normal Breathing" "Max Inhale Breath Hold" "Max Exhalation Breath Hold" "Plug Nose. Move air to chest" "Allow abdomen to relax." "Move air to abdomen." "Exhale Fully" "Inhale Fully" "Inhale Partially"] -> w550
          frame 0, Default {
          }
          frame 1 {
          }
          frame 2 {
          }
          frame 3 {
          }
          frame 4 {
          }
          frame 5 {
          }
          frame 6 {
          }
          frame 7 {
          }
          frame 8 {
          }
        }
        n248 = case "Next Instruction" shown="1" w551 {
          tunnel: ["Perform Normal Breathing" "Max Inhale Breath Hold" "Max Exhalation Breath Hold" "Plug Nose. Move air to chest" "Allow abdomen to relax." "Move air to abdomen." "Exhale Fully" "Inhale Fully" "Inhale Partially"] -> w552
          frame 0, Default {
          }
          frame 1 {
          }
          frame 2 {
          }
          frame 3 {
          }
          frame 4 {
          }
          frame 5 {
          }
          frame 6 {
          }
          frame 7 {
          }
          frame 8 {
          }
        }
      }
      frame "Routine 3" {
        w596 = 300.0  # Routine Time
        # "Supine Heart Monitoring"
        # "300"
        n249 = local read "Output"() -> (w591:bool)
        n250 = Not(x=w591) -> (.not. x?=w592:bool)
        n251 = call "Elapsed Time4"("Time Target (s)"=w596, "Reset"=w592) -> ("Get Start Time (s)"=w594:dbl, "Elapsed Time (s)"=w597:dbl, "Time has Elapsed"=w593:bool)  [unwired: 10 in, 5 out]
        n252 = script code="t = [0, 30, ... % BP 1\n       50, 60, 80, ... % max inhale hold\n       120, 110, 130, ...% max exhale hold\n        150, 160, 180, ... % tidal breath hold\n        240, 270, 300]; % BP 2\n\n\nevent =  [1, 0,  ...\n                0, 2, 0, ...\n                0, 3, 0, ...\n                0, 4, 0, ...\n                 1, 0, 0];\n\nfor i = 2:length(t)\n    if ((x>=t(i-1)) &&  (x<t(i)))\n        y = event(i-1);\n        yNext = event(i);\n       % dt = t(i) - t(i-1);\n        break;\n    end\nend" "Routine timing"("x"=w597) -> ("yNext"=w598:dbl, "y"=w601:dbl)  [unwired: 1 in, 1 out]
        n253 = property on="Total Routine Time" class="Slide (strict)"("Scale.Maximum"=w596) -> ()  [unwired: 2 in, 2 out]
        n254 = Seconds To Date/Time(time stamp (now)=w594) -> (date time rec=w595:T2)  [unwired: 1 in]
        n255 = case shown="True" w593 {
          frame False {
            # "Routine Not Done. Continue buffering."
            n256 = flat-sequence {
              frame #0 {
                w604 = FALSE
                w603 = TRUE
                n257 = local write "Stop Acquisition"(w604) -> ()
                n258 = local write "BIO Connect"(w604) -> ()
                n259 = local write "Play Sound"(w603) -> ()
                n260 = local write "Output"(w603) -> ()
                n261 = local write "Start Acquisition"(w603) -> ()
              }
              frame #1 {
                n262 = local write "Buffer"(TRUE) -> ()
              }
            }
          }
          frame True {
            # "Routine done. Save."
            n263 = flat-sequence {
              frame #0 {
                n264 = local write "Buffer"(FALSE) -> ()
              }
              frame #1 {
                n265 = local write "Play Sound"(FALSE) -> ()
                n266 = local write "Output"(FALSE) -> ()
                n267 = local write "Start Acquisition"(FALSE) -> ()
                n268 = local write "Stop Acquisition"(TRUE) -> ()
              }
              frame #2 {
                n269 = local write "Save"(TRUE) -> ()
              }
              frame #3 {
                n270 = Wait (ms)(milliseconds to wait=500) -> ()  [unwired: 1 out]
              }
              frame #4 {
                n271 = local write "Flush"(TRUE) -> ()
              }
              frame #5 {
                n272 = local write "Flush"(FALSE) -> ()
                n273 = local write "Save"(FALSE) -> ()
              }
              frame #6 {
                n274 = local write "Routine Selection"(enum16{"Default"}."Default") -> ()
              }
            }
          }
        }
        n275 = case shown="4" w601 {
          tunnel: ["Remain Still" "Begin Blood Pressure Recording" "Max Inhale Breath Hold" "Max Exhale Breath Hold" "Tidal Breath Hold"] -> w600
          frame 0, Default {
          }
          frame 1 {
          }
          frame 2 {
          }
          frame 3 {
          }
          frame 4 {
          }
        }
        n276 = case shown="4" w598 {
          tunnel: ["Remain Still" "Begin Blood Pressure Recording" "Max Inhale Breath Hold" "Max Exhale Breath Hold" "Tidal Breath Hold"] -> w599
          frame 0, Default {
          }
          frame 1 {
          }
          frame 2 {
          }
          frame 3 {
          }
          frame 4 {
          }
        }
      }
      frame "Routine 4" {
        w637 = 180.0  # Routine Time
        # "Seated Heart Monitoring"
        # "300"
        n277 = local read "Output"() -> (w630:bool)
        n278 = Not(x=w630) -> (.not. x?=w631:bool)
        n279 = call "Elapsed Time5"("Time Target (s)"=w637, "Reset"=w631) -> ("Get Start Time (s)"=w635:dbl, "Elapsed Time (s)"=w627:dbl, "Time has Elapsed"=w634:bool)  [unwired: 10 in, 5 out]
        n280 = script code="t = [0, 30, ... % BP 1\n       50, 60, 80, ... % max inhale hold\n       120, 110, 130, ...% max exhale hold\n        150, 160, 180, ... % tidal breath hold\n        240, 270, 300]; % BP 2\n\n\nevent =  [1, 0,  ...\n                0, 2, 0, ...\n                0, 3, 0, ...\n                0, 4, 0, ...\n                 1, 0, 0];\n\nfor i = 2:length(t)\n    if ((x>=t(i-1)) &&  (x<t(i)))\n        y = event(i-1);\n        yNext = event(i);\n       % dt = t(i) - t(i-1);\n        break;\n    end\nend" "Routine timing"("x"=w627) -> ("yNext"=w629:dbl, "y"=w628:dbl)  [unwired: 1 in, 1 out]
        n281 = property on="Total Routine Time" class="Slide (strict)"("Scale.Maximum"=w637) -> ()  [unwired: 2 in, 2 out]
        n282 = Seconds To Date/Time(time stamp (now)=w635) -> (date time rec=w636:T2)  [unwired: 1 in]
        n283 = case shown="False" w634 {
          frame False {
            # "Routine Not Done. Continue buffering."
            n284 = flat-sequence {
              frame #0 {
                w650 = FALSE
                w649 = TRUE
                n285 = local write "Play Sound"(w649) -> ()
                n286 = local write "Stop Acquisition"(w650) -> ()
                n287 = local write "Output"(w649) -> ()
                n288 = local write "Start Acquisition"(w649) -> ()
                n289 = local write "BIO Connect"(w650) -> ()
              }
              frame #1 {
                n290 = local write "Buffer"(TRUE) -> ()
              }
            }
          }
          frame True {
            # "Routine done. Save."
            n291 = flat-sequence {
              frame #0 {
                n292 = local write "Buffer"(FALSE) -> ()
              }
              frame #1 {
                w653 = FALSE
                n293 = local write "Play Sound"(w653) -> ()
                n294 = local write "Output"(w653) -> ()
                n295 = local write "Start Acquisition"(w653) -> ()
                n296 = local write "Stop Acquisition"(TRUE) -> ()
              }
              frame #2 {
                n297 = local write "Save"(TRUE) -> ()
              }
              frame #3 {
                n298 = Wait (ms)(milliseconds to wait=500) -> ()  [unwired: 1 out]
              }
              frame #4 {
                n299 = local write "Flush"(TRUE) -> ()
              }
              frame #5 {
                n300 = local write "Flush"(FALSE) -> ()
                n301 = local write "Save"(FALSE) -> ()
              }
              frame #6 {
                n302 = local write "Routine Selection"(enum16{"Default"}."Default") -> ()
              }
            }
          }
        }
        n303 = case shown="4" w628 {
          tunnel: ["Remain Still" "Begin Blood Pressure Recording" "Max Inhale Breath Hold" "Max Exhale Breath Hold" "Tidal Breath Hold"] -> w633
          frame 0, Default {
          }
          frame 1 {
          }
          frame 2 {
          }
          frame 3 {
          }
          frame 4 {
          }
        }
        n304 = case shown="4" w629 {
          tunnel: ["Remain Still" "Begin Blood Pressure Recording" "Max Inhale Breath Hold" "Max Exhale Breath Hold" "Tidal Breath Hold"] -> w632
          frame 0, Default {
          }
          frame 1 {
          }
          frame 2 {
          }
          frame 3 {
          }
          frame 4 {
          }
        }
      }
      frame "Routine 5a" {
        w664 = 300.0  # Routine Time
        # "Relaxation"
        # "240"
        n305 = local read "Output"() -> (w661:bool)
        n306 = Not(x=w661) -> (.not. x?=w662:bool)
        n307 = call "Elapsed Time7"("Time Target (s)"=w664, "Reset"=w662) -> ("Get Start Time (s)"=w666:dbl, "Elapsed Time (s)"=w665:dbl, "Time has Elapsed"=w663:bool)  [unwired: 10 in, 5 out]
        n308 = script code="t = [0, 30, 240, 270, 300];\n\n\nevent =  [1, 0, 1, 0, 0];\n\nfor i = 2:length(t)\n    if ((x>=t(i-1)) &&  (x<t(i)))\n        y = event(i-1);\n        yNext = event(i);\n       % dt = t(i) - t(i-1);\n        break;\n    end\nend" "Routine timing"("x"=w665) -> ("yNext"=w667:dbl, "y"=w668:dbl)  [unwired: 1 in, 1 out]
        n309 = property on="Total Routine Time" class="Slide (strict)"("Scale.Maximum"=w664) -> ()  [unwired: 2 in, 2 out]
        n310 = Seconds To Date/Time(time stamp (now)=w666) -> (date time rec=w672:T2)  [unwired: 1 in]
        n311 = case shown="False" w663 {
          frame False {
            n312 = flat-sequence {
              frame #0 {
                w673 = FALSE
                w674 = TRUE
                n313 = local write "Output"(w674) -> ()
                n314 = local write "Start Acquisition"(w674) -> ()
                n315 = local write "Play Sound"(w674) -> ()
                n316 = local write "Stop Acquisition"(w673) -> ()
                n317 = local write "BIO Connect"(w673) -> ()
              }
              frame #1 {
                n318 = local write "Buffer"(TRUE) -> ()
              }
            }
          }
          frame True {
            # "Routine done. Save."
            n319 = flat-sequence {
              frame #0 {
                n320 = local write "Buffer"(FALSE) -> ()
              }
              frame #1 {
                w678 = FALSE
                n321 = local write "Stop Acquisition"(TRUE) -> ()
                n322 = local write "Output"(w678) -> ()
                n323 = local write "Start Acquisition"(w678) -> ()
                n324 = local write "Play Sound"(w678) -> ()
              }
              frame #2 {
                n325 = local write "Save"(TRUE) -> ()
              }
              frame #3 {
                n326 = Wait (ms)(milliseconds to wait=500) -> ()  [unwired: 1 out]
              }
              frame #4 {
                n327 = local write "Flush"(TRUE) -> ()
              }
              frame #5 {
                n328 = local write "Flush"(FALSE) -> ()
                n329 = local write "Save"(FALSE) -> ()
              }
              frame #6 {
                n330 = local write "Routine Selection"(enum16{"Default"}."Default") -> ()
              }
            }
          }
        }
        n331 = case shown="0, Default" w668 {
          tunnel: ["Relax" "Begin Blood Pressure Recording"] -> w671
          frame 0, Default {
          }
          frame 1 {
          }
        }
        n332 = case shown="0, Default" w667 {
          tunnel: ["Relax" "Begin Blood Pressure Recording"] -> w670
          frame 0, Default {
          }
          frame 1 {
          }
        }
      }
      frame "Routine 5b" {
        w695 = 400.0  # Routine Time
        # "Attention"
        n333 = local read "Output"() -> (w689:bool)
        n334 = Not(x=w689) -> (.not. x?=w690:bool)
        n335 = call "Elapsed Time6"("Time Target (s)"=w695, "Reset"=w690) -> ("Get Start Time (s)"=w694:dbl, "Elapsed Time (s)"=w691:dbl, "Time has Elapsed"=w692:bool)  [unwired: 10 in, 5 out]
        n336 = script code="t = [0, 30, 240, 270, 300];\n\n\nevent =  [1, 0, 1, 0, 0];\n\nfor i = 2:length(t)\n    if ((x>=t(i-1)) &&  (x<t(i)))\n        y = event(i-1);\n        yNext = event(i);\n       % dt = t(i) - t(i-1);\n        break;\n    end\nend" "Routine timing"("x"=w691) -> ("yNext"=w697:dbl, "y"=w699:dbl)  [unwired: 1 in, 1 out]
        n337 = property on="Total Routine Time" class="Slide (strict)"("Scale.Maximum"=w695) -> ()  [unwired: 2 in, 2 out]
        n338 = Seconds To Date/Time(time stamp (now)=w694) -> (date time rec=w693:T2)  [unwired: 1 in]
        n339 = case shown="False" w692 {
          frame False {
            # "Routine Not Done. Continue buffering."
            n340 = flat-sequence {
              tunnel: "OpenHTML" -> [w704]
              frame #0 {
                w703 = FALSE
                w702 = TRUE
                n341 = case shown="True" w704 {
                  frame False {
                  }
                  frame True {
                    n342 = local write "OpenHTML"(FALSE) -> ()
                    n343 = call-poly <vilib>:"Open URL in Default Browser.vi"("URL"="\"C:\\Users\\tbc38\\Documents\\AttentionTest\\mackworth\\vigilanceTest.html\"") -> ()  [unwired: 5 in, 2 out]
                  }
                }
                n344 = local write "Stop Acquisition"(w703) -> ()
                n345 = local write "Play Sound"(w702) -> ()
                n346 = local write "Output"(w702) -> ()
                n347 = local write "Start Acquisition"(w702) -> ()
                n348 = local write "BIO Connect"(w703) -> ()
              }
              frame #1 {
                n349 = local write "Buffer"(TRUE) -> ()
              }
            }
          }
          frame True {
            # "Routine done. Save."
            n350 = flat-sequence {
              frame #0 {
                n351 = local write "Buffer"(FALSE) -> ()
              }
              frame #1 {
                w709 = FALSE
                n352 = local write "Play Sound"(w709) -> ()
                n353 = local write "Output"(w709) -> ()
                n354 = local write "Start Acquisition"(w709) -> ()
                n355 = local write "Stop Acquisition"(TRUE) -> ()
              }
              frame #2 {
                n356 = local write "Save"(TRUE) -> ()
              }
              frame #3 {
                n357 = Wait (ms)(milliseconds to wait=500) -> ()  [unwired: 1 out]
              }
              frame #4 {
                n358 = local write "Flush"(TRUE) -> ()
              }
              frame #5 {
                n359 = local write "Save"(FALSE) -> ()
                n360 = local write "Flush"(FALSE) -> ()
              }
              frame #6 {
                n361 = local write "Routine Selection"(enum16{"Default"}."Default") -> ()
              }
            }
          }
        }
        n362 = case shown="1" w699 {
          tunnel: ["Perform Attention Test" "Begin Blood Pressure Recording"] -> w698
          frame 0, Default {
          }
          frame 1 {
          }
        }
        n363 = case shown="1" w697 {
          tunnel: ["Perform Attention Test" "Begin Blood Pressure Recording"] -> w696
          frame 0, Default {
          }
          frame 1 {
          }
        }
      }
    }
    "Current Routine" <- w420
    "Current Instruction" <- w414
    "Next Instruction" <- w417
    "Total Routine Time" <- w415
    "Elapsed Time" <- w416
    "Start Time" <- w413
  }
  n364 = To Unsigned Long Integer(number=w3) -> (unsigned 32bit integer=w17:u32)
  n365 = Initialize Array(0.0, w4, w17) -> (w19:dbl[][])
  n366 = property class="niUSRP"(reference=w127, error in=w128, "Carrier Frequency"="Ch3&4 carrier frequency [Hz] 2", "Bandwidth"=5000000.0 ("Configuration:Bandwidth")) -> (reference out=w98:refnum<k15>, error out=w97:errorcluster)
  n367 = Obtain Queue(max queue size (-1, unlimited)=-1, name (unnamed)="BIOPAC View", element data type=w19) -> (queue out=w10:refnum<queue>)  [unwired: 2 in, 2 out]
  n368 = property class="niUSRP"(reference=w193, error in=w194, "Carrier Frequency"="Ch1&2 carrier frequency [Hz]", "Bandwidth"=5000000.0 ("Configuration:Bandwidth")) -> (reference out=w164:refnum<k15>, error out=w163:errorcluster)
  n369 = while {
    tunnel: w10 -> [w739]
    shift-right: [w733] -> _
    shift-left: dbl[] [] -> [w734]
    shift-right: [w731] -> _
    shift-left: dbl[] [] -> [w732]
    shift-right: [w730] -> _
    shift-left: dbl[] [] -> [w729]
    shift-right: [w727] -> _
    shift-left: dbl[] [] -> [w728]
    stop <- FALSE stop-if-true
    # "SHOW/VIEWING"
    n370 = local read "ACQ ms"() -> (w722:dbl)
    n371 = local read "Receiving"() -> (w721:bool)
    n372 = Get Queue Status(queue=w739) -> (# elements in queue=w737:i32)  [unwired: 2 in, 7 out]
    "# BIOViewQ2" <- w737
    n373 = Wait (ms)(milliseconds to wait=w722) -> ()  [unwired: 1 out]
    n374 = And(x="Show BIO", y=w721) -> (x .and. y?=w735:bool)
    n375 = case shown="True" w735 {
      tunnel: w739 -> [_ w754]
      tunnel: w737 -> [_ w753]
      tunnel: w734 -> [_ w751]
      tunnel: [w740 w750] -> w733
      tunnel: w732 -> [_ w748]
      tunnel: [w740 w747] -> w731
      tunnel: [w740 w746] -> w730
      tunnel: w729 -> [_ w744]
      tunnel: [w740 w743] -> w727
      tunnel: w728 -> [_ w741]
      frame False {
        w740 = dbl[] []
      }
      frame True {
        n376 = for {
          N: w753 -> [_]
          tunnel: [w763] -> w749 mode=concatenating
          tunnel: [w760] -> w745 mode=concatenating
          tunnel: [w759] -> w742 mode=concatenating
          tunnel: w754 -> [w756]
          tunnel: [w755] -> w752 mode=concatenating
          n377 = Dequeue Element(queue=w756) -> (element=w757:dbl[][])  [unwired: 2 in, 3 out]
          n378 = Index Array(array=w757, index (row)=0) -> (element=w759:dbl[])  [unwired: 1 in]
          n379 = Index Array(array=w757, index (row)=1) -> (element=w760:dbl[])  [unwired: 1 in]
          n380 = Index Array(array=w757, index (row)=2) -> (element=w763:dbl[])  [unwired: 1 in]
          n381 = Index Array(array=w757, index (row)=3) -> (element=w755:dbl[])  [unwired: 1 in]
        }
        n382 = Build Array (concatenate)(w741, w742) -> (w743:dbl[])
        n383 = Build Array (concatenate)(w744, w745) -> (w746:dbl[])
        n384 = Build Array (concatenate)(w748, w749) -> (w747:dbl[])
        n385 = Build Array (concatenate)(w751, w752) -> (w750:dbl[])
      }
    }
    "Array 1 View" <- w727
    "Array 2 View" <- w730
    "Array 3 View" <- w731
    "Array 4 View" <- w733
    n386 = local read "# ACQ cycles"() -> (w723:i32)
    n387 = Array Size(array=w727) -> (size(s)=w726:i32)
    "View Array Size" <- w726
    n388 = Divide(x=w726, y=w722) -> (x/y=w725:dbl)
    "# Elements in Array" <- w725
    n389 = Subtract(x=w723, y=w725) -> (x-y=→"ACQ -# Elements":dbl)
  }
  n390 = property class="niUSRP"(reference=w98, error in=w97, "Active Channel"="0", "Gain"="Rx2 Gain 1", "Active Antenna"=w85) -> (reference out=w102:refnum<k15>, error out=w101:errorcluster)
  n391 = property class="niUSRP" props=["Active Channel", "Gain", "Active Antenna", "Bandwidth"](reference=w164, error in=w163, "Active Channel"="0", "Gain"="Rx1 Gain 1", "Active Antenna"=w86) -> (reference out=w168:refnum<k15>, error out=w167:errorcluster)  [unwired: 1 out]
  n392 = To Unsigned Long Integer(number=w3) -> (unsigned 32bit integer=w6:u32)
  n393 = Initialize Array(0.0, w4, w6) -> (w8:dbl[][])
  n394 = Obtain Queue(max queue size (-1, unlimited)=-1, name (unnamed)="BIOPAC Buffer", element data type=w8) -> (queue out=w2:refnum<queue>)  [unwired: 2 in, 2 out]
  n395 = while {
    tunnel: w10 -> [w765]
    tunnel: w2 -> [w767]
    stop <- FALSE stop-if-true
    # "START ACQUISITION"
    n396 = local read "Connected"() -> (w772:bool)
    n397 = local read "Receiving"() -> (w770:bool)
    n398 = Not(x=w770) -> (.not. x?=w771:bool)
    n399 = And(x=w772, y=w771) -> (x .and. y?=w773:bool)
    n400 = And(x="Start Acquisition", y=w773) -> (x .and. y?=w774:bool)
    n401 = case shown="True" w774 {
      tunnel: w765 -> [_ w779]
      tunnel: w767 -> [_ w778]
      frame False {
      }
      frame True {
        n402 = flat-sequence {
          tunnel: [w784] -> w777
          tunnel: w777 -> [w788]
          tunnel: [w788] -> w776
          tunnel: w776 -> [w790]
          tunnel: [w790] -> w780
          tunnel: w780 -> [w793]
          tunnel: w779 -> [w792]
          tunnel: w778 -> [w791]
          frame #0 {
            n403 = dll-call lib="C:/Program Files (x86)/BIOPAC Systems, Inc/BIOPAC Hardware API 2.2 Education/x64/mpdev.dll" fn="startMPAcqDaemon" label="start Acq Daemon"() -> ()  [unwired: 4 in, 2 out]
            n404 = local write "Start Acquisition"(FALSE) -> ()
            n405 = local write "Stop Acquisition"(FALSE) -> ()
            n406 = local write "Receiving"(TRUE) -> ()
          }
          frame #1 {
            w785 = u32 1  # MPSUCCESS
            n407 = dll-call lib="C:/Program Files (x86)/BIOPAC Systems, Inc/BIOPAC Hardware API 2.2 Education/x64/mpdev.dll" fn="startAcquisition" label="start Acquisition"() -> ("return type"=w786:u32)  [unwired: 3 in, 2 out]
            n408 = Equal?(x=w786, y=w785) -> (x = y?=w784:bool)
          }
          frame #2 {
            n409 = local write "Acq Started"(TRUE) -> ()
          }
          frame #3 {
            n410 = local read "ACQ ms"() -> (w789:dbl)
            n411 = Wait (ms)(milliseconds to wait=w789) -> ()  [unwired: 1 out]
          }
          frame #4 {
            n412 = local read "Sample Rate"() -> (w798:dbl)
            n413 = local read "# Channels"() -> (w796:dbl)
            n414 = local read "ACQ ms"() -> (w797:dbl)
            n415 = Reciprocal(x=w798) -> (1/x=w801:dbl)
            n416 = Multiply(x=w801, y=w797) -> (x*y=w799:dbl)
            n417 = Multiply(x=w799, y=w796) -> (x*y=w794:dbl)
            "Receive Total Size" <- w794
            n418 = Initialize Array(0.0, w794) -> (w795:dbl[])
            n419 = case shown="True" w793 {
              tunnel: w795 -> [_ w806]
              tunnel: w794 -> [_ w805]
              tunnel: w792 -> [_ w804]
              tunnel: w791 -> [_ w802]
              frame False {
              }
              frame True {
                n420 = while {
                  tunnel: w806 -> [w832]
                  tunnel: w805 -> [w831]
                  tunnel: w804 -> [w807]
                  shift-right: [w818] -> _
                  shift-left: 0 -> [w819]
                  tunnel: w802 -> [w811]
                  stop <- w814 stop-if-true
                  w829 = u32 1  # MPSUCCESS
                  n421 = Add(x=w819, y=1) -> (x+y=w818:i32)
                  "# ACQ cycles" <- w818
                  n422 = dll-call lib="C:/Program Files (x86)/BIOPAC Systems, Inc/BIOPAC Hardware API 2.2 Education/x64/mpdev.dll" fn="receiveMPData"("value"=w832, "bytetoread"=w831, "bytesread"=0) -> ("return type"=w830:i32, "value"=w824:dbl[], "bytetoread"=→"Bytes To Read":u32, "bytesread"=→"Bytes Read":i32)  [unwired: 3 in, 2 out]
                  n423 = Decimate 1D Array(w824) -> (w825:dbl[], w826:dbl[], w827:dbl[], w823:dbl[])
                  n424 = Equal?(x=w830, y=w829) -> (x = y?=w813:bool)
                  n425 = Build Array(w825, w826, w827, w823) -> (w808:dbl[][])
                  n426 = local read "Show BIO"() -> (w809:bool)
                  n427 = local write "Receive Success"(w813) -> ()
                  n428 = case shown="True" w809 {
                    tunnel: w808 -> [_ w834]
                    tunnel: w807 -> [_ w833]
                    frame False {
                    }
                    frame True {
                      n429 = Enqueue Element(queue=w833, element=w834) -> ()  [unwired: 2 in, 3 out]
                    }
                  }
                  n430 = local read "Buffer"() -> (w812:bool)
                  n431 = case shown="True" w812 {
                    tunnel: w808 -> [_ w836]
                    tunnel: w811 -> [_ w835]
                    frame False {
                    }
                    frame True {
                      n432 = Enqueue Element(queue=w835, element=w836) -> ()  [unwired: 2 in, 3 out]
                    }
                  }
                  n433 = Get Queue Status(queue=w811) -> (# elements in queue=w810:i32)  [unwired: 2 in, 7 out]
                  n434 = local write "# BIO Buffer"(w810) -> ()
                  n435 = local read "Stop Acquisition"() -> (w814:bool)
                  n436 = local read "ACQ ms"() -> (w815:dbl)
                  n437 = Subtract(x=w815, y=0.0) -> (x-y=w822:dbl)
                  n438 = Wait (ms)(milliseconds to wait=w822) -> ()  [unwired: 1 out]
                }
              }
            }
          }
          frame #5 {
            n439 = local write "Receiving"(FALSE) -> ()
            n440 = local write "Acq Started"(FALSE) -> ()
          }
        }
      }
    }
    n441 = Get Queue Status(queue=w765) -> (# elements in queue=→"# BIO View Q":i32)  [unwired: 2 in, 7 out]
    n442 = Get Queue Status(queue=w767) -> (# elements in queue=→"# BIO Buffer":i32)  [unwired: 2 in, 7 out]
  }
  n443 = property class="niUSRP"(reference=w102, error in=w101, "Active Channel"="1", "Gain"="Rx2 Gain 2", "Active Antenna"=w85) -> (reference out=w130:refnum<k15>, error out=w129:errorcluster)
  n444 = call <instrlib>:"niUSRP Open Tx Session.vi"("device names"=w150, "error in (no error)"=w129) -> ("session handle out"=w137:refnum<k15>, "error out"=w136:errorcluster)  [unwired: 12 in]
  n445 = property class="niUSRP"(reference=w137, error in=w136, "Enabled Channels"="0,1" ("Configuration:Enabled Channels")) -> (reference out=w125:refnum<k15>, error out=w124:errorcluster)
  n446 = property class="niUSRP"(reference=w125, error in=w124, "IQ Rate"="Tx IQ Rate 2") -> (reference out=w119:refnum<k15>, error out=w120:errorcluster, "IQ Rate"=w118:dbl)
  n447 = property class="niUSRP" props=["Model", "Reference Frequency Source", "Timebase Clock Source"](reference=w119, error in=w120, "Reference Frequency Source"="RefIn" ("Clocking and Synchronization:Reference Frequency Source"), "Timebase Clock Source"="PpsIn" ("Clocking and Synchronization:Timebase Clock Source")) -> (reference out=w121:refnum<k15>, error out=w122:errorcluster)  [unwired: 1 out]
  n448 = property class="niUSRP"(reference=w121, error in=w122, "Carrier Frequency"="Ch3&4 carrier frequency [Hz] 2") -> (reference out=w92:refnum<k15>, error out=w91:errorcluster)
  n449 = property class="niUSRP"(reference=w92, error in=w91, "Active Channel"="0", "Gain"="Tx2 Gain 1", "Active Antenna"=w114) -> (reference out=w96:refnum<k15>, error out=w95:errorcluster)
  n450 = property class="niUSRP"(reference=w96, error in=w95, "Active Channel"="1", "Gain"="Tx2 Gain 2", "Active Antenna"=w114) -> (reference out=w116:refnum<k15>, error out=w117:errorcluster)
  n451 = property class="niUSRP"(reference=w168, error in=w167, "Active Channel"="1", "Gain"="Rx1 Gain 2", "Active Antenna"=w86) -> (reference out=w196:refnum<k15>, error out=w195:errorcluster)
  n452 = call <instrlib>:"niUSRP Open Tx Session.vi"("device names"=w216, "error in (no error)"=w195) -> ("session handle out"=w203:refnum<k15>, "error out"=w202:errorcluster)  [unwired: 12 in]
  n453 = property class="niUSRP"(reference=w203, error in=w202, "Enabled Channels"="0,1" ("Configuration:Enabled Channels")) -> (reference out=w191:refnum<k15>, error out=w190:errorcluster)
  n454 = property class="niUSRP"(reference=w191, error in=w190, "IQ Rate"="Tx IQ Rate 1") -> (reference out=w185:refnum<k15>, error out=w186:errorcluster, "IQ Rate"=w184:dbl)
  n455 = property class="niUSRP" props=["Model", "Reference Frequency Source", "Timebase Clock Source"](reference=w185, error in=w186, "Reference Frequency Source"="RefIn" ("Clocking and Synchronization:Reference Frequency Source"), "Timebase Clock Source"="PpsIn" ("Clocking and Synchronization:Timebase Clock Source")) -> (reference out=w187:refnum<k15>, error out=w188:errorcluster)  [unwired: 1 out]
  n456 = property class="niUSRP"(reference=w187, error in=w188, "Carrier Frequency"="Ch1&2 carrier frequency [Hz]") -> (reference out=w158:refnum<k15>, error out=w157:errorcluster)
  n457 = property class="niUSRP"(reference=w158, error in=w157, "Active Channel"="0", "Gain"="Tx1 Gain 1", "Active Antenna"=w180) -> (reference out=w162:refnum<k15>, error out=w161:errorcluster)
  n458 = property class="niUSRP"(reference=w162, error in=w161, "Active Channel"="1", "Gain"="Tx1 Gain 2", "Active Antenna"=w180) -> (reference out=w182:refnum<k15>, error out=w183:errorcluster)
  n459 = while {
    stop <- FALSE stop-if-true
    # "DISCONNECT"
    n460 = Wait (ms)(milliseconds to wait=500) -> ()  [unwired: 1 out]
    n461 = case shown="True" "Disconnect" {
      frame False {
      }
      frame True {
        w842 = FALSE
        n462 = dll-call lib="C:/Program Files (x86)/BIOPAC Systems, Inc/BIOPAC Hardware API 2.2 Education/x64/mpdev.dll" fn="disconnectMPDev" label="disconnect"() -> ()  [unwired: 4 in, 2 out]
        n463 = local write "Disconnect"(w842) -> ()
        n464 = local write "Disconnected"(TRUE) -> ()
        n465 = local write "Connected"(w842) -> ()
      }
    }
  }
  n466 = while {
    stop <- FALSE stop-if-true
    n467 = local read "Output"() -> (w845:bool)
    n468 = Wait (ms)(milliseconds to wait=10.0) -> ()  [unwired: 1 out]
    n469 = case shown="True" w845 {
      tunnel: [w851 "Channel 1 Tone Amplitude"] -> w849
      tunnel: [w851 "Channel 2 Tone Amplitude"] -> w848
      tunnel: [w851 "Channel 3 Tone Amplitude"] -> w847
      tunnel: [w851 "Channel 4 Tone Amplitude"] -> w846
      frame False {
        w851 = 0.0 ("Channel 1\nTone Amplitude")
      }
      frame True {
      }
    }
    "Ch1 Amplitude" <- w849
    "Ch2 Amplitude" <- w848
    "Ch3 Amplitude" <- w847
    "Ch4 Amplitude" <- w846
  }
  n470 = call <instrlib>:"niUSRP Commit.vi"("session handle"=w116, "error in (no error)"=w117) -> ("session handle out"=w152:refnum<k15>, "error out"=w153:errorcluster)  [unwired: 12 in]
  n471 = call <instrlib>:"niUSRP Commit.vi"("session handle"=w182, "error in (no error)"=w183) -> ("session handle out"=w218:refnum<k15>, "error out"=w219:errorcluster)  [unwired: 12 in]
  n472 = Merge Errors(w129, w153) -> (w144:errorcluster)
  n473 = Merge Errors(w195, w219) -> (w210:errorcluster)
  n474 = call <instrlib>:"niUSRP Set Time.vi"("session handle"=w130, "apply timestamp"=w142, "timestamp"=T4 {"whole seconds"=0, "fractional seconds"=0.0}, "error in (no error)"=w144) -> ("session handle out"=w146:refnum<k15>, "error out"=w145:errorcluster)  [unwired: 10 in]
  n475 = call <instrlib>:"niUSRP Initiate.vi"("session handle"=w146, "error in (no error)"=w145) -> ("session handle out"=w156:refnum<k15>, "error out"=w84:errorcluster)  [unwired: 12 in]
  n476 = while {
    tunnel: w118 -> [w866]
    tunnel: w84 -> [w861]
    stop <- FALSE stop-if-true
    # "Generate I and Q waveforms."
    n477 = Bundle By Name(cluster=cluster{"Fs":dbl, "#s":dbl} {"Fs"=1000.0, "#s"=1000.0} ("sampling info"), "Fs"=w866, "#s"="Waveform Size 2") -> (w867:cluster{"Fs":dbl, "#s":dbl})
    n478 = Wait (ms)(milliseconds to wait=u32 500) -> ()  [unwired: 1 out]
    n479 = local read "Ch3 Amplitude"() -> (w857:dbl)
    n480 = local read "Ch4 Amplitude"() -> (w856:dbl)
    n481 = call <vilib>:"Sine Waveform.vi"("sampling info"=w867, "error in (no error)"=w861, "phase"=90.0, "amplitude"=w857, "frequency"="Channel 3 Tone Frequency") -> ("error out"=w862:errorcluster, "signal out"=w880:waveform(dbl))  [unwired: 5 in]
    n482 = call <vilib>:"Sine Waveform.vi"("sampling info"=w867, "error in (no error)"=w861, "amplitude"=w857, "frequency"="Channel 3 Tone Frequency") -> ("error out"=w863:errorcluster, "signal out"=w881:waveform(dbl))  [unwired: 6 in]
    n483 = call <vilib>:"Sine Waveform.vi"("sampling info"=w867, "error in (no error)"=w861, "phase"=90.0, "amplitude"=w856, "frequency"="Channel 4 Tone Frequency") -> ("error out"=w864:errorcluster, "signal out"=w871:waveform(dbl))  [unwired: 5 in]
    n484 = call <vilib>:"Sine Waveform.vi"("sampling info"=w867, "error in (no error)"=w861, "amplitude"=w856, "frequency"="Channel 4 Tone Frequency") -> ("error out"=w865:errorcluster, "signal out"=w870:waveform(dbl))  [unwired: 6 in]
    n485 = Merge Errors(w862, w863, w864, w865) -> ()  [unwired: 1 out]
    n486 = Build Array(w880, w881, w871, w870) -> (→"Tx2 Waveform Graph":waveform(dbl)[])
    n487 = Unbundle By Name(w880) -> ("Y"=w879:dbl[])
    n488 = Unbundle By Name(w881) -> ("Y"=w878:dbl[])
    n489 = Unbundle By Name(w871) -> ("Y"=w874:dbl[])
    n490 = Unbundle By Name(w870) -> ("Y"=w873:dbl[])
    n491 = Re/Im To Complex(1:w878, 2:w879) -> (0:w869:cdb[])
    n492 = Re/Im To Complex(1:w873, 2:w874) -> (0:w868:cdb[])
    n493 = Build Array(w869, w868) -> (→"Tx2 Waveform":cdb[][])
  }
  n494 = call <instrlib>:"niUSRP Set Time.vi"("session handle"=w196, "apply timestamp"=w208, "timestamp"=T4 {"whole seconds"=0, "fractional seconds"=0.0}, "error in (no error)"=w210) -> ("session handle out"=w212:refnum<k15>, "error out"=w211:errorcluster)  [unwired: 10 in]
  n495 = call <instrlib>:"niUSRP Initiate.vi"("session handle"=w212, "error in (no error)"=w211) -> ("session handle out"=w222:refnum<k15>, "error out"=w83:errorcluster)  [unwired: 12 in]
  n496 = while {
    tunnel: w184 -> [w895]
    tunnel: w83 -> [w887]
    stop <- FALSE stop-if-true
    # "Generate I and Q waveforms."
    n497 = Wait (ms)(milliseconds to wait=u32 500) -> ()  [unwired: 1 out]
    n498 = Bundle By Name(cluster=cluster{"Fs":dbl, "#s":dbl} {"Fs"=1000.0, "#s"=1000.0} ("sampling info"), "Fs"=w895, "#s"="Waveform Size 1") -> (w896:cluster{"Fs":dbl, "#s":dbl})
    n499 = local read "Ch1 Amplitude"() -> (w886:dbl)
    n500 = local read "Ch2 Amplitude"() -> (w885:dbl)
    n501 = call <vilib>:"Sine Waveform.vi"("sampling info"=w896, "error in (no error)"=w887, "phase"=90.0, "amplitude"=w886, "frequency"="Channel 1 Tone Frequency") -> ("error out"=w891:errorcluster, "signal out"=w909:waveform(dbl))  [unwired: 5 in]
    n502 = call <vilib>:"Sine Waveform.vi"("sampling info"=w896, "error in (no error)"=w887, "amplitude"=w886, "frequency"="Channel 1 Tone Frequency") -> ("error out"=w892:errorcluster, "signal out"=w910:waveform(dbl))  [unwired: 6 in]
    n503 = call <vilib>:"Sine Waveform.vi"("sampling info"=w896, "error in (no error)"=w887, "phase"=90.0, "amplitude"=w885, "frequency"="Channel 2 Tone Frequency") -> ("error out"=w893:errorcluster, "signal out"=w900:waveform(dbl))  [unwired: 5 in]
    n504 = call <vilib>:"Sine Waveform.vi"("sampling info"=w896, "error in (no error)"=w887, "amplitude"=w885, "frequency"="Channel 2 Tone Frequency") -> ("error out"=w894:errorcluster, "signal out"=w899:waveform(dbl))  [unwired: 6 in]
    n505 = Merge Errors(w891, w892, w893, w894) -> ()  [unwired: 1 out]
    n506 = Build Array(w909, w910, w900, w899) -> (→"Tx1 Waveform Graph":waveform(dbl)[])
    n507 = Unbundle By Name(w909) -> ("Y"=w908:dbl[])
    n508 = Unbundle By Name(w910) -> ("Y"=w907:dbl[])
    n509 = Unbundle By Name(w900) -> ("Y"=w903:dbl[])
    n510 = Unbundle By Name(w899) -> ("Y"=w902:dbl[])
    n511 = Re/Im To Complex(1:w907, 2:w908) -> (0:w898:cdb[])
    n512 = Re/Im To Complex(1:w902, 2:w903) -> (0:w897:cdb[])
    n513 = Build Array(w898, w897) -> (→"Tx1 Waveform":cdb[][])
  }
  n514 = local read "Waveform Size 2"() -> (w63:dbl)
  n515 = local read "Waveform Size 1"() -> (w73:dbl)
  n516 = Initialize Array(cdb 0.0+0.0i ("element"), 2 ("dimension size"), w63) -> (w65:cdb[][])
  n517 = Obtain Queue(max queue size (-1, unlimited)=-1, name (unnamed)="Rx2Queue", element data type=w65) -> (queue out=w61:refnum<queue>)  [unwired: 2 in, 2 out]
  n518 = Initialize Array(cdb 0.0+0.0i ("element"), 2 ("dimension size"), w73) -> (w70:cdb[][])
  n519 = while {
    tunnel: w61 -> [w914]
    stop <- FALSE stop-if-true
    n520 = Wait (ms)(milliseconds to wait=u32 200) -> ()  [unwired: 1 out]
    n521 = case shown="True" "Dis2" {
      tunnel: w914 -> [_ w920]
      frame False {
        n522 = Wait (ms)(milliseconds to wait=u32 500) -> ()  [unwired: 1 out]
      }
      frame True {
        n523 = Preview Queue Element(queue=w920) -> (element=w921:cdb[][])  [unwired: 2 in, 3 out]
        n524 = for {
          tunnel: w921 -> [w927] mode=indexing
          shift-right: [w924] -> w919
          shift-left: dbl[][] [] -> [w923]
          n525 = Complex To Re/Im(x + iy=w927) -> (x=w926:dbl[], y=w925:dbl[])
          n526 = Build Array (concatenate)(w923, w926, w925) -> (w924:dbl[][])
        }
        "IQ Graph 2" <- w919
      }
    }
  }
  n527 = while {
    tunnel: w156 -> [w938]
    tunnel: w84 -> [w937]
    tunnel: [w933] -> w111
    tunnel: [w936] -> w108
    shift-right: [w928] -> _
    shift-left: w61 -> [w929]
    stop <- w932 stop-if-true
    # "Rx on both channels"
    n528 = local read "Waveform Size 2"() -> (w931:dbl)
    n529 = call-poly <instrlib>:"niUSRP Fetch Rx Data (poly).vi"("session handle"=w938, "number of samples"=w931, "error in (no error)"=w937) -> ("session handle out"=w936:refnum<k15>, "data"=w930:cdb[][], "error out"=w933:errorcluster)  [unwired: 9 in, 1 out]
    n530 = Enqueue Element(queue=w929, element=w930) -> (queue out=w928:refnum<queue>)  [unwired: 2 in, 2 out]
    n531 = Unbundle By Name(w933) -> ("status"=w935:bool)
    n532 = Or(x=w935, y="Stop 2") -> (x .or. y?=w932:bool)
  }
  n533 = Obtain Queue(max queue size (-1, unlimited)=-1, name (unnamed)="Rx1Queue", element data type=w70) -> (queue out=w62:refnum<queue>)  [unwired: 2 in, 2 out]
  n534 = while {
    tunnel: w152 -> [w946]
    tunnel: w84 -> [w945]
    tunnel: [w943] -> w113
    tunnel: [w941] -> w106
    stop <- w942 stop-if-true
    # "Tx on both channels"
    n535 = local read "Tx2 Waveform"() -> (w939:cdb[][])
    n536 = local read "Stop 2"() -> (w940:bool)
    n537 = call-poly <instrlib>:"niUSRP Write Tx Data (poly).vi"("session handle"=w946, "data"=w939, "end of data?"=w940, "error in (no error)"=w945) -> ("session handle out"=w941:refnum<k15>, "error out"=w943:errorcluster)  [unwired: 10 in]
    n538 = Unbundle By Name(w943) -> ("status"=w944:bool)
    n539 = Compound Arithmetic op=OR(w944, w940) -> (w942:bool)
  }
  n540 = while {
    tunnel: w62 -> [w948]
    stop <- FALSE stop-if-true
    n541 = Wait (ms)(milliseconds to wait=u32 200) -> ()  [unwired: 1 out]
    n542 = case shown="True" "Dis1" {
      tunnel: w948 -> [_ w952]
      frame False {
        n543 = Wait (ms)(milliseconds to wait=u32 500) -> ()  [unwired: 1 out]
      }
      frame True {
        n544 = Preview Queue Element(queue=w952) -> (element=w954:cdb[][])  [unwired: 2 in, 3 out]
        n545 = for {
          tunnel: w954 -> [w960] mode=indexing
          shift-right: [w957] -> w953
          shift-left: dbl[][] [] -> [w956]
          n546 = Complex To Re/Im(x + iy=w960) -> (x=w959:dbl[], y=w958:dbl[])
          n547 = Build Array (concatenate)(w956, w959, w958) -> (w957:dbl[][])
        }
        "IQ Graph" <- w953
      }
    }
  }
  n548 = while {
    tunnel: w222 -> [w971]
    tunnel: w83 -> [w970]
    tunnel: [w966] -> w177
    tunnel: [w969] -> w174
    shift-right: [w961] -> _
    shift-left: w62 -> [w963]
    stop <- w965 stop-if-true
    # "Rx on both channels"
    n549 = local read "Waveform Size 1"() -> (w964:dbl)
    n550 = call-poly <instrlib>:"niUSRP Fetch Rx Data (poly).vi"("session handle"=w971, "number of samples"=w964, "error in (no error)"=w970) -> ("session handle out"=w969:refnum<k15>, "data"=w962:cdb[][], "error out"=w966:errorcluster)  [unwired: 9 in, 1 out]
    n551 = Enqueue Element(queue=w963, element=w962) -> (queue out=w961:refnum<queue>)  [unwired: 2 in, 2 out]
    n552 = Unbundle By Name(w966) -> ("status"=w968:bool)
    n553 = Or(x=w968, y="Stop") -> (x .or. y?=w965:bool)
  }
  n554 = while {
    tunnel: w218 -> [w979]
    tunnel: w83 -> [w978]
    tunnel: [w976] -> w179
    tunnel: [w974] -> w172
    stop <- w975 stop-if-true
    # "Tx on both channels"
    n555 = local read "Tx1 Waveform"() -> (w972:cdb[][])
    n556 = local read "Stop"() -> (w973:bool)
    n557 = call-poly <instrlib>:"niUSRP Write Tx Data (poly).vi"("session handle"=w979, "data"=w972, "end of data?"=w973, "error in (no error)"=w978) -> ("session handle out"=w974:refnum<k15>, "error out"=w976:errorcluster)  [unwired: 10 in]
    n558 = Unbundle By Name(w976) -> ("status"=w977:bool)
    n559 = Compound Arithmetic op=OR(w977, w973) -> (w975:bool)
  }
  n560 = flat-sequence {
    tunnel: [w981] -> w112
    tunnel: w113 -> [w981]
    tunnel: [w980] -> w107
    tunnel: w106 -> [w980]
    frame #0 {
      n561 = local write "Stop 2"(TRUE ("STOP")) -> ()
    }
  }
  n562 = flat-sequence {
    tunnel: [w984] -> w178
    tunnel: w179 -> [w984]
    tunnel: [w983] -> w173
    tunnel: w172 -> [w983]
    frame #0 {
      n563 = local write "Stop"(TRUE ("STOP")) -> ()
    }
  }
  n564 = flat-sequence {
    tunnel: [w987] -> w110
    tunnel: w111 -> [w987]
    tunnel: [w986] -> w109
    tunnel: w108 -> [w986]
    frame #0 {
      n565 = local write "Stop 2"(TRUE ("STOP")) -> ()
    }
  }
  n566 = flat-sequence {
    tunnel: [w990] -> w176
    tunnel: w177 -> [w990]
    tunnel: [w989] -> w175
    tunnel: w174 -> [w989]
    frame #0 {
      n567 = local write "Stop"(TRUE ("STOP")) -> ()
    }
  }
  n568 = local read "Rx IQ Rate 1"() -> (w40:dbl)
  n569 = call <instrlib>:"niUSRP Abort.vi"("session handle"=w109, "error in (no error)"=w110) -> ("session handle out"=w149:refnum<k15>, "error out"=w148:errorcluster)  [unwired: 12 in]
  n570 = local read "Waveform Size 1"() -> (w54:dbl)
  n571 = local read "DownSamplingRatio"() -> (w53:i32)
  n572 = call <instrlib>:"niUSRP Close Session.vi"("session handle"=w149, "error in (no error)"=w148) -> ("error out"=w105:errorcluster)  [unwired: 13 in]
  n573 = call <instrlib>:"niUSRP Close Session.vi"("session handle"=w107, "error in (no error)"=w112) -> ("error out"=w104:errorcluster)  [unwired: 13 in]
  n574 = Divide(x=w40, y="DownSamplingRatio1") -> (x/y=→"Sampling Rate":dbl)
  n575 = Divide(x=2000.0, y=2.0) -> (x/y=→"BW/2":dbl)
  n576 = call <instrlib>:"niUSRP Abort.vi"("session handle"=w175, "error in (no error)"=w176) -> ("session handle out"=w215:refnum<k15>, "error out"=w214:errorcluster)  [unwired: 12 in]
  n577 = flat-sequence {
    tunnel: w105 -> [w994]
    tunnel: w104 -> [w993]
    tunnel: [w992] -> w103
    frame #0 {
      n578 = Merge Errors(w994, w993) -> (w992:errorcluster)
      n579 = local write "Stop 2"(FALSE ("STOP")) -> ()
    }
  }
  n580 = Divide(x=w54, y=w53) -> (x/y=w32:dbl)
  n581 = call <instrlib>:"niUSRP Close Session.vi"("session handle"=w215, "error in (no error)"=w214) -> ("error out"=w171:errorcluster)  [unwired: 13 in]
  n582 = call <instrlib>:"niUSRP Close Session.vi"("session handle"=w173, "error in (no error)"=w178) -> ("error out"=w170:errorcluster)  [unwired: 13 in]
  n583 = flat-sequence {
    tunnel: w171 -> [w998]
    tunnel: w170 -> [w997]
    tunnel: [w996] -> w169
    frame #0 {
      n584 = Merge Errors(w998, w997) -> (w996:errorcluster)
      n585 = local write "Stop"(FALSE ("STOP")) -> ()
    }
  }
  n586 = Initialize Array(0.0 ("element"), w33, w32) -> (w55:dbl[][])
  n587 = Initialize Array(0.0 ("element"), w33, w32) -> (w42:dbl[][])
  n588 = Obtain Queue(name (unnamed)="Buffer", element data type=w42) -> (queue out=w41:refnum<queue>)  [unwired: 3 in, 2 out]
  n589 = Obtain Queue(name (unnamed)="ChsQueue", element data type=w55) -> (queue out=w52:refnum<queue>)  [unwired: 3 in, 2 out]
  n590 = while {
    tunnel: w62 -> [w1200]
    tunnel: w61 -> [w1197]
    tunnel: w52 -> [w1157]
    tunnel: w41 -> [w1155]
    tunnel: w2 -> [w1007]
    stop <- FALSE stop-if-true
    w1001 = 2 ("order")
    w1030 = Filter_Passband_Type."Bandpass" ("filter type")
    w1060 = Filter_Passband_Type."Bandpass" ("filter type")
    w1000 = Filter_Passband_Type."Bandpass" ("filter type")
    w1100 = Filter_Passband_Type."Bandpass" ("filter type")
    w1002 = 2 ("order")
    # "Tx4 to Rx4 QueInd_15"
    # "Tx3 to Rx4 QueInd_14"
    # "Tx2 to Rx4 QueInd_13"
    # "Tx1 to Rx4 QueInd_12"
    # "Tx4 to Rx3 QueInd_11"
    # "Tx3 to Rx3 QueInd_10"
    # "Tx2 to Rx3 QueInd_9"
    # "Tx1 to Rx3 QueInd_8"
    # "Tx1 to Rx4 QueInd_12"
    # "Tx2 to Rx4 QueInd_13"
    # "Tx2 to Rx3 QueInd_9"
    # "Tx1 to Rx3 QueInd_8"
    # "Tx4 to Rx2 QueInd_7"
    # "Tx3 to Rx2 QueInd_6"
    # "Tx4 to Rx1 QueInd_3"
    # "Tx3 to Rx1 QueInd_2"
    # "Tx4 to Rx2 QueInd_7"
    # "Tx4 to Rx4 QueInd_15"
    # "Tx3 to Rx2 QueInd_6"
    # "Tx4 to Rx3 QueInd_11"
    # "Tx2 to Rx2 QueInd_5"
    # "Tx2 to Rx2 QueInd_5"
    # "Tx1 to Rx2 QueInd_4"
    # "Tx4 to Rx1 QueInd_3"
    # "Tx3 to Rx1 QueInd_2"
    # "Tx2 to Rx1 QueInd_1"
    # "Tx1 to Rx1 QueInd_0"
    # "Tx2 to Rx1 QueInd_1"
    # "Tx3 to Rx4 QueInd_14"
    # "Tx3 to Rx3 QueInd_10"
    # "Tx1 to Rx2 QueInd_4"
    # "Tx1 to Rx1 QueInd_0"
    # "100 times"
    n591 = Dequeue Element(queue=w1200) -> (element=w1202:cdb[][])  [unwired: 2 in, 3 out]
    n592 = Get Queue Status(queue=w1200) -> (# elements in queue=→"# IQ queue Ch 1":i32)  [unwired: 2 in, 7 out]
    n593 = Get Queue Status(queue=w1197) -> (# elements in queue=→"# IQ queue Ch 2":i32)  [unwired: 2 in, 7 out]
    n594 = Dequeue Element(queue=w1197) -> (element=w1194:cdb[][])  [unwired: 2 in, 3 out]
    n595 = Index Array(array=w1202, index (row)=1) -> (element=w1083:cdb[])  [unwired: 1 in]
    n596 = Index Array(array=w1202, index (row)=0) -> (element=w1103:cdb[])  [unwired: 1 in]
    n597 = Index Array(array=w1194, index (row)=1) -> (element=w1036:cdb[])  [unwired: 1 in]
    n598 = Index Array(array=w1194, index (row)=0) -> (element=w1003:cdb[])  [unwired: 1 in]
    n599 = local read "Channel 2 Tone Frequency"() -> (w1142:dbl)
    n600 = local read "Channel 1 Tone Frequency"() -> (w1154:dbl)
    n601 = local read "Channel 3 Tone Frequency"() -> (w1084:dbl)
    n602 = local read "Channel 4 Tone Frequency"() -> (w1071:dbl)
    n603 = local read "Channel 4 Tone Frequency"() -> (w1102:dbl)
    n604 = local read "Channel 3 Tone Frequency"() -> (w1175:dbl)
    n605 = local read "Channel 3 Tone Frequency"() -> (w1113:dbl)
    n606 = local read "Channel 4 Tone Frequency"() -> (w1122:dbl)
    n607 = local read "Channel 2 Tone Frequency"() -> (w1149:dbl)
    n608 = local read "Channel 2 Tone Frequency"() -> (w1029:dbl)
    n609 = local read "Channel 1 Tone Frequency"() -> (w1191:dbl)
    n610 = local read "Channel 1 Tone Frequency"() -> (w1042:dbl)
    n611 = local read "Rx IQ Rate 1"() -> (w1104:dbl)
    n612 = local read "Channel 1 Tone Frequency"() -> (w1067:dbl)
    n613 = local read "Channel 2 Tone Frequency"() -> (w1047:dbl)
    n614 = local read "Channel 3 Tone Frequency"() -> (w1180:dbl)
    n615 = local read "Channel 4 Tone Frequency"() -> (w1133:dbl)
    n616 = local read "Rx IQ Rate 2"() -> (w1035:dbl)
    n617 = local read "BW/2"() -> (w1101:dbl)
    n618 = local read "BW/2"() -> (w1074:dbl)
    n619 = local read "Rx IQ Rate 1"() -> (w1082:dbl)
    n620 = local read "Rx IQ Rate 2"() -> (w1050:dbl)
    n621 = local read "BW/2"() -> (w1037:dbl)
    n622 = local read "BW/2"() -> (w1048:dbl)
    n623 = Subtract(x=w1084, y=w1074) -> (x-y=w1088:dbl)
    n624 = Subtract(x=w1102, y=w1101) -> (x-y=w1106:dbl)
    n625 = Subtract(x=w1142, y=w1074) -> (x-y=w1140:dbl)
    n626 = Add(x=w1084, y=w1074) -> (x+y=w1089:dbl)
    n627 = Add(x=w1071, y=w1074) -> (x+y=w1072:dbl)
    n628 = Subtract(x=w1071, y=w1074) -> (x-y=w1073:dbl)
    n629 = Subtract(x=w1029, y=w1037) -> (x-y=w1034:dbl)
    n630 = Subtract(x=w1191, y=w1101) -> (x-y=w1192:dbl)
    n631 = Add(x=w1102, y=w1101) -> (x+y=w1107:dbl)
    n632 = Add(x=w1142, y=w1074) -> (x+y=w1141:dbl)
    n633 = Subtract(x=w1149, y=w1101) -> (x-y=w1150:dbl)
    n634 = Subtract(x=w1113, y=w1101) -> (x-y=w1114:dbl)
    n635 = Subtract(x=w1042, y=w1037) -> (x-y=w1043:dbl)
    n636 = Add(x=w1029, y=w1037) -> (x+y=w1033:dbl)
    n637 = Add(x=w1191, y=w1101) -> (x+y=w1193:dbl)
    n638 = Add(x=w1149, y=w1101) -> (x+y=w1151:dbl)
    n639 = Add(x=w1113, y=w1101) -> (x+y=w1115:dbl)
    n640 = Add(x=w1042, y=w1037) -> (x+y=w1044:dbl)
    n641 = Subtract(x=w1154, y=w1074) -> (x-y=w1187:dbl)
    n642 = Add(x=w1154, y=w1074) -> (x+y=w1188:dbl)
    n643 = Subtract(x=w1122, y=w1037) -> (x-y=w1123:dbl)
    n644 = Add(x=w1122, y=w1037) -> (x+y=w1124:dbl)
    n645 = Subtract(x=w1175, y=w1037) -> (x-y=w1178:dbl)
    n646 = Add(x=w1175, y=w1037) -> (x+y=w1179:dbl)
    n647 = Subtract(x=w1067, y=w1048) -> (x-y=w1066:dbl)
    n648 = Subtract(x=w1133, y=w1048) -> (x-y=w1131:dbl)
    n649 = Add(x=w1067, y=w1048) -> (x+y=w1065:dbl)
    n650 = Add(x=w1133, y=w1048) -> (x+y=w1132:dbl)
    n651 = Subtract(x=w1047, y=w1048) -> (x-y=w1049:dbl)
    n652 = Subtract(x=w1180, y=w1048) -> (x-y=w1183:dbl)
    n653 = Add(x=w1047, y=w1048) -> (x+y=w1051:dbl)
    n654 = Add(x=w1180, y=w1048) -> (x+y=w1184:dbl)
    n655 = call-poly <vilib>:"Butterworth Filter.vi"("init/cont (init:F)"=TRUE, "order"=w1002, "filter type"=w1100, "low cutoff freq: fl"=w1106, "high cutoff freq: fh"=w1107, "sampling freq: fs"=w1104, "X"=w1103) -> ("Filtered X"=w1099:cdb[])  [unwired: 1 in, 1 out]
    n656 = call-poly <vilib>:"Butterworth Filter.vi"("init/cont (init:F)"=TRUE, "order"=w1002, "filter type"=w1100, "low cutoff freq: fl"=w1150, "high cutoff freq: fh"=w1151, "sampling freq: fs"=w1104, "X"=w1103) -> ("Filtered X"=w1148:cdb[])  [unwired: 1 in, 1 out]
    n657 = call-poly <vilib>:"Butterworth Filter.vi"("init/cont (init:F)"=TRUE, "order"=w1002, "filter type"=w1100, "low cutoff freq: fl"=w1114, "high cutoff freq: fh"=w1115, "sampling freq: fs"=w1104, "X"=w1103) -> ("Filtered X"=w1112:cdb[])  [unwired: 1 in, 1 out]
    n658 = call-poly <vilib>:"Butterworth Filter.vi"("init/cont (init:F)"=TRUE, "order"=w1002, "filter type"=w1100, "low cutoff freq: fl"=w1192, "high cutoff freq: fh"=w1193, "sampling freq: fs"=w1104, "X"=w1103) -> ("Filtered X"=w1190:cdb[])  [unwired: 1 in, 1 out]
    n659 = call-poly <vilib>:"Butterworth Filter.vi"("init/cont (init:F)"=TRUE, "order"=w1002, "filter type"=w1000, "low cutoff freq: fl"=w1187, "high cutoff freq: fh"=w1188, "sampling freq: fs"=w1082, "X"=w1083) -> ("Filtered X"=w1186:cdb[])  [unwired: 1 in, 1 out]
    n660 = call-poly <vilib>:"Butterworth Filter.vi"("init/cont (init:F)"=TRUE, "order"=w1001, "filter type"=w1030, "low cutoff freq: fl"=w1034, "high cutoff freq: fh"=w1033, "sampling freq: fs"=w1035, "X"=w1036) -> ("Filtered X"=w1031:cdb[])  [unwired: 1 in, 1 out]
    n661 = call-poly <vilib>:"Butterworth Filter.vi"("init/cont (init:F)"=TRUE, "order"=w1002, "filter type"=w1000, "low cutoff freq: fl"=w1088, "high cutoff freq: fh"=w1089, "sampling freq: fs"=w1082, "X"=w1083) -> ("Filtered X"=w1087:cdb[])  [unwired: 1 in, 1 out]
    n662 = call-poly <vilib>:"Butterworth Filter.vi"("init/cont (init:F)"=TRUE, "order"=w1002, "filter type"=w1000, "low cutoff freq: fl"=w1073, "high cutoff freq: fh"=w1072, "sampling freq: fs"=w1082, "X"=w1083) -> ("Filtered X"=w1080:cdb[])  [unwired: 1 in, 1 out]
    n663 = call-poly <vilib>:"Butterworth Filter.vi"("init/cont (init:F)"=TRUE, "order"=w1001, "filter type"=w1030, "low cutoff freq: fl"=w1043, "high cutoff freq: fh"=w1044, "sampling freq: fs"=w1035, "X"=w1036) -> ("Filtered X"=w1046:cdb[])  [unwired: 1 in, 1 out]
    n664 = call-poly <vilib>:"Butterworth Filter.vi"("init/cont (init:F)"=TRUE, "order"=w1002, "filter type"=w1000, "low cutoff freq: fl"=w1140, "high cutoff freq: fh"=w1141, "sampling freq: fs"=w1082, "X"=w1083) -> ("Filtered X"=w1139:cdb[])  [unwired: 1 in, 1 out]
    n665 = call-poly <vilib>:"Butterworth Filter.vi"("init/cont (init:F)"=TRUE, "order"=w1001, "filter type"=w1030, "low cutoff freq: fl"=w1123, "high cutoff freq: fh"=w1124, "sampling freq: fs"=w1035, "X"=w1036) -> ("Filtered X"=w1121:cdb[])  [unwired: 1 in, 1 out]
    n666 = call-poly <vilib>:"Butterworth Filter.vi"("init/cont (init:F)"=TRUE, "order"=w1001, "filter type"=w1030, "low cutoff freq: fl"=w1178, "high cutoff freq: fh"=w1179, "sampling freq: fs"=w1035, "X"=w1036) -> ("Filtered X"=w1177:cdb[])  [unwired: 1 in, 1 out]
    n667 = call-poly <vilib>:"Butterworth Filter.vi"("init/cont (init:F)"=TRUE, "order"=w1001, "filter type"=w1060, "low cutoff freq: fl"=w1066, "high cutoff freq: fh"=w1065, "sampling freq: fs"=w1050, "X"=w1003) -> ("Filtered X"=w1069:cdb[])  [unwired: 1 in, 1 out]
    n668 = call-poly <vilib>:"Butterworth Filter.vi"("init/cont (init:F)"=TRUE, "order"=w1001, "filter type"=w1060, "low cutoff freq: fl"=w1049, "high cutoff freq: fh"=w1051, "sampling freq: fs"=w1050, "X"=w1003) -> ("Filtered X"=w1059:cdb[])  [unwired: 1 in, 1 out]
    n669 = call-poly <vilib>:"Butterworth Filter.vi"("init/cont (init:F)"=TRUE, "order"=w1001, "filter type"=w1060, "low cutoff freq: fl"=w1131, "high cutoff freq: fh"=w1132, "sampling freq: fs"=w1050, "X"=w1003) -> ("Filtered X"=w1130:cdb[])  [unwired: 1 in, 1 out]
    n670 = call-poly <vilib>:"Butterworth Filter.vi"("init/cont (init:F)"=TRUE, "order"=w1001, "filter type"=w1060, "low cutoff freq: fl"=w1183, "high cutoff freq: fh"=w1184, "sampling freq: fs"=w1050, "X"=w1003) -> ("Filtered X"=w1182:cdb[])  [unwired: 1 in, 1 out]
    n671 = Complex To Polar(r * e^(i*theta)=w1099) -> (r=w1098:dbl[])  [unwired: 1 out]
    n672 = Complex To Polar(r * e^(i*theta)=w1112) -> (r=w1110:dbl[])  [unwired: 1 out]
    n673 = Complex To Polar(r * e^(i*theta)=w1148) -> (r=w1147:dbl[])  [unwired: 1 out]
    n674 = Complex To Polar(r * e^(i*theta)=w1190) -> (r=w1174:dbl[])  [unwired: 1 out]
    n675 = Complex To Polar(r * e^(i*theta)=w1087) -> (r=w1086:dbl[])  [unwired: 1 out]
    n676 = Complex To Polar(r * e^(i*theta)=w1080) -> (r=w1079:dbl[])  [unwired: 1 out]
    n677 = Complex To Polar(r * e^(i*theta)=w1186) -> (r=w1161:dbl[])  [unwired: 1 out]
    n678 = Complex To Polar(r * e^(i*theta)=w1139) -> (r=w1138:dbl[])  [unwired: 1 out]
    n679 = local read "DownSamplingRatio"() -> (w1076:i32)
    n680 = local read "DownSamplingRatio"() -> (w1093:i32)
    n681 = Complex To Polar(r * e^(i*theta)=w1069) -> (r=w1068:dbl[])  [unwired: 1 out]
    n682 = Complex To Polar(r * e^(i*theta)=w1059) -> (r=w1058:dbl[])  [unwired: 1 out]
    n683 = Complex To Polar(r * e^(i*theta)=w1182) -> (r=w1160:dbl[])  [unwired: 1 out]
    n684 = Complex To Polar(r * e^(i*theta)=w1130) -> (r=w1129:dbl[])  [unwired: 1 out]
    n685 = Complex To Polar(r * e^(i*theta)=w1031) -> (r=w1023:dbl[])  [unwired: 1 out]
    n686 = Complex To Polar(r * e^(i*theta)=w1046) -> (r=w1039:dbl[])  [unwired: 1 out]
    n687 = local read "Waveform Size 1"() -> (w1096:dbl)
    n688 = Complex To Polar(r * e^(i*theta)=w1177) -> (r=w1159:dbl[])  [unwired: 1 out]
    n689 = Complex To Polar(r * e^(i*theta)=w1121) -> (r=w1120:dbl[])  [unwired: 1 out]
    n690 = local read "DownSamplingRatio"() -> (w1025:i32)
    n691 = local read "DownSamplingRatio"() -> (w1054:i32)
    n692 = local read "Waveform Size 1"() -> (w1077:dbl)
    n693 = local read "Waveform Size 2"() -> (w1056:dbl)
    n694 = local read "Waveform Size 2"() -> (w1026:dbl)
    n695 = Divide(x=w1077, y=w1076) -> (x/y=w1085:dbl)
    n696 = Divide(x=w1077, y=w1076) -> (x/y=w1078:dbl)
    n697 = Divide(x=w1077, y=w1076) -> (x/y=w1137:dbl)
    n698 = Divide(x=w1096, y=w1093) -> (x/y=w1097:dbl)
    n699 = Divide(x=w1096, y=w1093) -> (x/y=w1146:dbl)
    n700 = Divide(x=w1096, y=w1093) -> (x/y=w1111:dbl)
    n701 = Divide(x=w1096, y=w1093) -> (x/y=w1173:dbl)
    n702 = Divide(x=w1077, y=w1076) -> (x/y=w1162:dbl)
    n703 = Divide(x=w1056, y=w1054) -> (x/y=w1062:dbl)
    n704 = Divide(x=w1026, y=w1025) -> (x/y=w1119:dbl)
    n705 = Divide(x=w1056, y=w1054) -> (x/y=w1057:dbl)
    n706 = Divide(x=w1056, y=w1054) -> (x/y=w1128:dbl)
    n707 = Divide(x=w1026, y=w1025) -> (x/y=w1024:dbl)
    n708 = Reshape Array(w1086, w1085, w1076) -> (w1091:dbl[][])
    n709 = Divide(x=w1056, y=w1054) -> (x/y=w1168:dbl)
    n710 = Reshape Array(w1079, w1078, w1076) -> (w1061:dbl[][])
    n711 = Divide(x=w1026, y=w1025) -> (x/y=w1040:dbl)
    n712 = Divide(x=w1026, y=w1025) -> (x/y=w1165:dbl)
    n713 = Reshape Array(w1138, w1137, w1076) -> (w1136:dbl[][])
    n714 = Reshape Array(w1098, w1097, w1093) -> (w1095:dbl[][])
    n715 = Reshape Array(w1110, w1111, w1093) -> (w1109:dbl[][])
    n716 = Reshape Array(w1174, w1173, w1093) -> (w1172:dbl[][])
    n717 = Reshape Array(w1161, w1162, w1076) -> (w1170:dbl[][])
    n718 = Reshape Array(w1147, w1146, w1093) -> (w1145:dbl[][])
    n719 = Reshape Array(w1068, w1062, w1054) -> (w1064:dbl[][])
    n720 = Reshape Array(w1120, w1119, w1025) -> (w1118:dbl[][])
    n721 = Reshape Array(w1058, w1057, w1054) -> (w1055:dbl[][])
    n722 = Reshape Array(w1129, w1128, w1054) -> (w1127:dbl[][])
    n723 = Reshape Array(w1023, w1024, w1025) -> (w1028:dbl[][])
    n724 = Reshape Array(w1160, w1168, w1054) -> (w1167:dbl[][])
    n725 = Reshape Array(w1039, w1040, w1025) -> (w1041:dbl[][])
    n726 = Reshape Array(w1159, w1165, w1025) -> (w1164:dbl[][])
    n727 = for {
      tunnel: w1172 -> [w1243] mode=indexing
      tunnel: [w1242] -> w1171 mode=indexing
      workers-P: _ -> [_]
      n728 = Add Array Elements(numeric array=w1243) -> (sum=w1242:dbl)
    }
    n729 = for {
      tunnel: w1145 -> [w1228] mode=indexing
      tunnel: [w1227] -> w1144 mode=indexing
      workers-P: _ -> [_]
      n730 = Add Array Elements(numeric array=w1228) -> (sum=w1227:dbl)
    }
    n731 = for {
      tunnel: w1109 -> [w1220] mode=indexing
      tunnel: [w1219] -> w1108 mode=indexing
      workers-P: _ -> [_]
      n732 = Add Array Elements(numeric array=w1220) -> (sum=w1219:dbl)
    }
    n733 = for {
      tunnel: w1095 -> [w1218] mode=indexing
      tunnel: [w1217] -> w1094 mode=indexing
      workers-P: _ -> [_]
      n734 = Add Array Elements(numeric array=w1218) -> (sum=w1217:dbl)
    }
    n735 = for {
      tunnel: w1091 -> [w1216] mode=indexing
      tunnel: [w1215] -> w1092 mode=indexing
      workers-P: _ -> [_]
      n736 = Add Array Elements(numeric array=w1216) -> (sum=w1215:dbl)
    }
    n737 = for {
      tunnel: w1170 -> [w1241] mode=indexing
      tunnel: [w1240] -> w1169 mode=indexing
      workers-P: _ -> [_]
      n738 = Add Array Elements(numeric array=w1241) -> (sum=w1240:dbl)
    }
    n739 = for {
      tunnel: w1061 -> [w1214] mode=indexing
      tunnel: [w1213] -> w1075 mode=indexing
      workers-P: _ -> [_]
      n740 = Add Array Elements(numeric array=w1214) -> (sum=w1213:dbl)
    }
    n741 = for {
      tunnel: w1136 -> [w1226] mode=indexing
      tunnel: [w1225] -> w1135 mode=indexing
      workers-P: _ -> [_]
      n742 = Add Array Elements(numeric array=w1226) -> (sum=w1225:dbl)
    }
    n743 = for {
      tunnel: w1064 -> [w1212] mode=indexing
      tunnel: [w1211] -> w1063 mode=indexing
      workers-P: _ -> [_]
      n744 = Add Array Elements(numeric array=w1212) -> (sum=w1211:dbl)
    }
    n745 = for {
      tunnel: w1055 -> [w1210] mode=indexing
      tunnel: [w1209] -> w1053 mode=indexing
      workers-P: _ -> [_]
      n746 = Add Array Elements(numeric array=w1210) -> (sum=w1209:dbl)
    }
    n747 = for {
      tunnel: w1127 -> [w1224] mode=indexing
      tunnel: [w1223] -> w1126 mode=indexing
      workers-P: _ -> [_]
      n748 = Add Array Elements(numeric array=w1224) -> (sum=w1223:dbl)
    }
    n749 = for {
      tunnel: w1028 -> [w1206] mode=indexing
      tunnel: [w1205] -> w1027 mode=indexing
      workers-P: _ -> [_]
      n750 = Add Array Elements(numeric array=w1206) -> (sum=w1205:dbl)
    }
    n751 = for {
      tunnel: w1167 -> [w1239] mode=indexing
      tunnel: [w1238] -> w1166 mode=indexing
      workers-P: _ -> [_]
      n752 = Add Array Elements(numeric array=w1239) -> (sum=w1238:dbl)
    }
    n753 = for {
      tunnel: w1041 -> [w1208] mode=indexing
      tunnel: [w1207] -> w1038 mode=indexing
      workers-P: _ -> [_]
      n754 = Add Array Elements(numeric array=w1208) -> (sum=w1207:dbl)
    }
    n755 = for {
      tunnel: w1164 -> [w1237] mode=indexing
      tunnel: [w1236] -> w1163 mode=indexing
      workers-P: _ -> [_]
      n756 = Add Array Elements(numeric array=w1237) -> (sum=w1236:dbl)
    }
    n757 = for {
      tunnel: w1118 -> [w1222] mode=indexing
      tunnel: [w1221] -> w1117 mode=indexing
      workers-P: _ -> [_]
      n758 = Add Array Elements(numeric array=w1222) -> (sum=w1221:dbl)
    }
    n759 = Divide(x=w1092, y=w1076) -> (x/y=w1017:dbl[])
    n760 = Divide(x=w1075, y=w1076) -> (x/y=w1016:dbl[])
    n761 = Divide(x=w1135, y=w1076) -> (x/y=w1018:dbl[])
    n762 = Divide(x=w1171, y=w1093) -> (x/y=w1158:dbl[])
    n763 = Divide(x=w1169, y=w1076) -> (x/y=w1019:dbl[])
    n764 = Divide(x=w1144, y=w1093) -> (x/y=w1022:dbl[])
    n765 = Divide(x=w1108, y=w1093) -> (x/y=w1021:dbl[])
    n766 = Divide(x=w1094, y=w1093) -> (x/y=w1020:dbl[])
    n767 = Divide(x=w1063, y=w1054) -> (x/y=w1015:dbl[])
    n768 = Divide(x=w1053, y=w1054) -> (x/y=w1014:dbl[])
    n769 = Divide(x=w1166, y=w1054) -> (x/y=w1013:dbl[])
    n770 = Divide(x=w1126, y=w1054) -> (x/y=w1012:dbl[])
    n771 = Divide(x=w1027, y=w1025) -> (x/y=w1009:dbl[])
    n772 = Divide(x=w1163, y=w1025) -> (x/y=w1010:dbl[])
    n773 = Divide(x=w1038, y=w1025) -> (x/y=w1008:dbl[])
    n774 = Divide(x=w1117, y=w1025) -> (x/y=w1011:dbl[])
    n775 = Build Array(w1158, w1022, w1021, w1020, w1019, w1018, w1017, w1016, w1015, w1014, w1013, w1012, w1008, w1009, w1010, w1011) -> (w1156:dbl[][])
    "ChAmp" <- w1156
    n776 = local read "Acq Started"() -> (w1004:bool)
    n777 = local read "Buffer"() -> (w1005:bool)
    n778 = local read "Flush"() -> (w1153:bool)
    n779 = And(x=w1004, y=w1005) -> (x .and. y?=w1006:bool)
    n780 = case shown="True" w1006 {
      tunnel: w1155 -> [w1231 w1235]
      tunnel: w1156 -> [_ w1234]
      tunnel: w1153 -> [w1230 _]
      tunnel: w1007 -> [w1229 _]
      frame False {
        n781 = case shown="True" w1230 {
          tunnel: w1231 -> [_ w1233]
          tunnel: w1229 -> [_ w1232]
          frame False {
          }
          frame True {
            n782 = Flush Queue(queue=w1232) -> ()  [unwired: 1 in, 3 out]
            n783 = Flush Queue(queue=w1233) -> ()  [unwired: 1 in, 3 out]
          }
        }
      }
      frame True {
        n784 = Enqueue Element(queue=w1235, element=w1234) -> ()  [unwired: 2 in, 3 out]
      }
    }
    n785 = Enqueue Element(queue=w1157, element=w1156) -> ()  [unwired: 2 in, 3 out]
  }
  n786 = local read "DownSamplingRatio"() -> (w50:i32)
  n787 = local read "Waveform Size 1"() -> (w51:dbl)
  n788 = Divide(x=w51, y=w50) -> (x/y=w37:dbl)
  n789 = Divide(x=w37, y="DownSamplingRatio 2") -> (x/y=w28:dbl)
  n790 = Multiply(x=w27, y=w28) -> (x*y=w45:dbl)
  n791 = Initialize Array(w26, w27, w28) -> (w49:dbl[][])
  n792 = Initialize Array(w26, w27, w28) -> (w48:dbl[][])
  n793 = Initialize Array(w26, w27, w28) -> (w47:dbl[][])
  n794 = Initialize Array(w26, w27, w28) -> (w46:dbl[][])
  n795 = Initialize Array(w26, w27, w28) -> (w25:dbl[][])
  n796 = Initialize Array(w26, w27, w28) -> (w24:dbl[][])
  n797 = Initialize Array(w26, w27, w28) -> (w23:dbl[][])
  n798 = Initialize Array(w26, w27, w28) -> (w22:dbl[][])
  n799 = while {
    tunnel: w27 -> [w1357]
    tunnel: w52 -> [w1350]
    shift-right: [w1347] -> _
    shift-left: w49 -> [w1329]
    tunnel: w45 -> [w1265]
    shift-right: [w1341] -> _
    shift-left: w48 -> [w1353]
    shift-right: [w1340] -> _
    shift-left: w47 -> [w1352]
    shift-right: [w1339] -> _
    shift-left: w46 -> [w1351]
    tunnel: "DownSamplingRatio 2" -> [w1280]
    tunnel: w28 -> [w1289]
    tunnel: "DownSamplingRatio 2" -> [w1313]
    shift-right: [w1261] -> _
    shift-left: w25 -> [w1275]
    shift-right: [w1260] -> _
    shift-left: w24 -> [w1267]
    shift-right: [w1259] -> _
    shift-left: w23 -> [w1270]
    shift-right: [w1258] -> _
    shift-left: w22 -> [w1277]
    stop <- FALSE stop-if-true
    # "Tx4 to Rx4 QueInd_15"
    # "Tx3 to Rx4 QueInd_14"
    # "Tx2 to Rx4 QueInd_13"
    # "Tx1 to Rx4 QueInd_12"
    # "Tx4 to Rx3 QueInd_11"
    # "Tx3 to Rx3 QueInd_10"
    # "Tx2 to Rx3 QueInd_9"
    # "Tx1 to Rx3 QueInd_8"
    # "Tx4 to Rx2 QueInd_7"
    # "Tx3 to Rx2 QueInd_6"
    # "Tx2 to Rx2 QueInd_5"
    # "Tx1 to Rx2 QueInd_4"
    # "Tx4 to Rx1 QueInd_3"
    # "Tx3 to Rx1 QueInd_2"
    # "Tx2 to Rx1 QueInd_1"
    # "Tx1 to Rx1 QueInd_0"
    n800 = local read "Sampling Rate"() -> (w1314:dbl)
    n801 = Get Queue Status(queue=w1350) -> (# elements in queue=→"# elements in view queue":i32)  [unwired: 2 in, 7 out]
    n802 = Dequeue Element(queue=w1350) -> (element=w1294:dbl[][])  [unwired: 2 in, 3 out]
    n803 = Decrement(x=w1357) -> (x-1=w1268:i32)
    n804 = Divide(x=w1314, y=w1313) -> (x/y=→"Dis Sampling Rate":dbl)
    n805 = Index Array(array=w1294, index (row)=10 ("index")) -> (element=w1293:dbl[])  [unwired: 1 in]
    n806 = Index Array(array=w1294, index (row)=11 ("index")) -> (element=w1292:dbl[])  [unwired: 1 in]
    n807 = Index Array(array=w1294, index (row)=15 ("index")) -> (element=w1291:dbl[])  [unwired: 1 in]
    n808 = Index Array(array=w1294, index (row)=14 ("index")) -> (element=w1290:dbl[])  [unwired: 1 in]
    n809 = Index Array(array=w1294, index (row)=0 ("index")) -> (element=w1327:dbl[])  [unwired: 1 in]
    n810 = Index Array(array=w1294, index (row)=1 ("index")) -> (element=w1326:dbl[])  [unwired: 1 in]
    n811 = Index Array(array=w1294, index (row)=5 ("index")) -> (element=w1325:dbl[])  [unwired: 1 in]
    n812 = Index Array(array=w1294, index (row)=4 ("index")) -> (element=w1324:dbl[])  [unwired: 1 in]
    n813 = Array Subset(array=w1270, index (row)=0 ("index"), length (row)=w1268) -> (w1269:dbl[][])  [unwired: 2 in]
    n814 = Array Subset(array=w1277, index (row)=0 ("index"), length (row)=w1268) -> (w1276:dbl[][])  [unwired: 2 in]
    n815 = Array Subset(array=w1267, index (row)=0 ("index"), length (row)=w1268) -> (w1266:dbl[][])  [unwired: 2 in]
    n816 = Array Subset(array=w1275, index (row)=0 ("index"), length (row)=w1268) -> (w1274:dbl[][])  [unwired: 2 in]
    n817 = Array Subset(array=w1329, index (row)=0 ("index"), length (row)=w1268) -> (w1348:dbl[][])  [unwired: 2 in]
    n818 = Array Subset(array=w1353, index (row)=0 ("index"), length (row)=w1268) -> (w1344:dbl[][])  [unwired: 2 in]
    n819 = Array Subset(array=w1352, index (row)=0 ("index"), length (row)=w1268) -> (w1343:dbl[][])  [unwired: 2 in]
    n820 = Array Subset(array=w1351, index (row)=0 ("index"), length (row)=w1268) -> (w1342:dbl[][])  [unwired: 2 in]
    n821 = Reshape Array(w1292, w1289, w1280) -> (w1287:dbl[][])
    n822 = Reshape Array(w1291, w1289, w1280) -> (w1286:dbl[][])
    n823 = Reshape Array(w1290, w1289, w1280) -> (w1285:dbl[][])
    n824 = Reshape Array(w1326, w1289, w1280) -> (w1321:dbl[][])
    n825 = Reshape Array(w1325, w1289, w1280) -> (w1320:dbl[][])
    n826 = Reshape Array(w1324, w1289, w1280) -> (w1319:dbl[][])
    n827 = Reshape Array(w1293, w1289, w1280) -> (w1288:dbl[][])
    n828 = Reshape Array(w1327, w1289, w1280) -> (w1323:dbl[][])
    n829 = for {
      tunnel: w1286 -> [w1367] mode=indexing
      tunnel: [w1366] -> w1282 mode=indexing
      workers-P: _ -> [_]
      n830 = Add Array Elements(numeric array=w1367) -> (sum=w1366:dbl)
    }
    n831 = for {
      tunnel: w1285 -> [w1365] mode=indexing
      tunnel: [w1364] -> w1281 mode=indexing
      workers-P: _ -> [_]
      n832 = Add Array Elements(numeric array=w1365) -> (sum=w1364:dbl)
    }
    n833 = for {
      tunnel: w1320 -> [w1375] mode=indexing
      tunnel: [w1374] -> w1317 mode=indexing
      workers-P: _ -> [_]
      n834 = Add Array Elements(numeric array=w1375) -> (sum=w1374:dbl)
    }
    n835 = for {
      tunnel: w1319 -> [w1373] mode=indexing
      tunnel: [w1372] -> w1316 mode=indexing
      workers-P: _ -> [_]
      n836 = Add Array Elements(numeric array=w1373) -> (sum=w1372:dbl)
    }
    n837 = for {
      tunnel: w1287 -> [w1369] mode=indexing
      tunnel: [w1368] -> w1283 mode=indexing
      workers-P: _ -> [_]
      n838 = Add Array Elements(numeric array=w1369) -> (sum=w1368:dbl)
    }
    n839 = for {
      tunnel: w1321 -> [w1377] mode=indexing
      tunnel: [w1376] -> w1318 mode=indexing
      workers-P: _ -> [_]
      n840 = Add Array Elements(numeric array=w1377) -> (sum=w1376:dbl)
    }
    n841 = for {
      tunnel: w1288 -> [w1371] mode=indexing
      tunnel: [w1370] -> w1284 mode=indexing
      workers-P: _ -> [_]
      n842 = Add Array Elements(numeric array=w1371) -> (sum=w1370:dbl)
    }
    n843 = for {
      tunnel: w1323 -> [w1379] mode=indexing
      tunnel: [w1378] -> w1322 mode=indexing
      workers-P: _ -> [_]
      n844 = Add Array Elements(numeric array=w1379) -> (sum=w1378:dbl)
    }
    n845 = Divide(x=w1284, y=w1280) -> (x/y=w1249:dbl[])
    n846 = Divide(x=w1322, y=w1280) -> (x/y=w1251:dbl[])
    n847 = Divide(x=w1283, y=w1280) -> ()  [unwired: 1 out]
    n848 = Divide(x=w1282, y=w1280) -> (x/y=w1248:dbl[])
    n849 = Divide(x=w1318, y=w1280) -> ()  [unwired: 1 out]
    n850 = Divide(x=w1317, y=w1280) -> (x/y=w1250:dbl[])
    n851 = Divide(x=w1281, y=w1280) -> ()  [unwired: 1 out]
    n852 = Divide(x=w1316, y=w1280) -> ()  [unwired: 1 out]
    n853 = Build Array (concatenate)(w1248, w1269) -> (w1259:dbl[][])
    n854 = Build Array (concatenate)(w1248, w1276) -> (w1258:dbl[][])
    n855 = Build Array (concatenate)(w1249, w1266) -> (w1260:dbl[][])
    n856 = Build Array (concatenate)(w1249, w1274) -> (w1261:dbl[][])
    n857 = Build Array (concatenate)(w1250, w1342) -> (w1339:dbl[][])
    n858 = Build Array (concatenate)(w1250, w1343) -> (w1340:dbl[][])
    n859 = Build Array (concatenate)(w1251, w1344) -> (w1341:dbl[][])
    n860 = Build Array (concatenate)(w1251, w1348) -> (w1347:dbl[][])
    n861 = Reshape Array(w1259, w1265) -> (w1263:dbl[])
    n862 = Reshape Array(w1258, w1265) -> (w1262:dbl[])
    n863 = Reshape Array(w1260, w1265) -> (w1264:dbl[])
    n864 = Reshape Array(w1261, w1265) -> (w1273:dbl[])
    n865 = Reshape Array(w1339, w1265) -> (w1300:dbl[])
    n866 = Reshape Array(w1340, w1265) -> (w1301:dbl[])
    n867 = Reshape Array(w1341, w1265) -> (w1302:dbl[])
    n868 = Reshape Array(w1347, w1265) -> (w1303:dbl[])
    n869 = local read "Dis Sampling Rate"() -> (w1304:dbl)
    n870 = call-poly <vilib>:"Butterworth Filter.vi"("init/cont (init:F)"=TRUE, "order"=3, "filter type"="top filter", "low cutoff freq: fl"="fl Top", "high cutoff freq: fh"="fh Top", "sampling freq: fs"=w1304, "X"=w1303) -> ("Filtered X"=w1299:dbl[])  [unwired: 1 in, 1 out]
    n871 = call-poly <vilib>:"Butterworth Filter.vi"("init/cont (init:F)"=TRUE, "order"=3, "filter type"="bottom filter", "low cutoff freq: fl"="fl Bottom", "high cutoff freq: fh"="fh Bottom", "sampling freq: fs"=w1304, "X"=w1302) -> ("Filtered X"=w1332:dbl[])  [unwired: 1 in, 1 out]
    n872 = call-poly <vilib>:"Butterworth Filter.vi"("init/cont (init:F)"=TRUE, "order"=3, "filter type"="top filter", "low cutoff freq: fl"="fl Top", "high cutoff freq: fh"="fh Top", "sampling freq: fs"=w1304, "X"=w1273) -> ("Filtered X"=w1257:dbl[])  [unwired: 1 in, 1 out]
    n873 = call-poly <vilib>:"Butterworth Filter.vi"("init/cont (init:F)"=TRUE, "order"=3, "filter type"="bottom filter", "low cutoff freq: fl"="fl Bottom", "high cutoff freq: fh"="fh Bottom", "sampling freq: fs"=w1304, "X"=w1264) -> ("Filtered X"=w1256:dbl[])  [unwired: 1 in, 1 out]
    n874 = call-poly <vilib>:"Butterworth Filter.vi"("init/cont (init:F)"=TRUE, "order"=3, "filter type"="top filter", "low cutoff freq: fl"="fl Top", "high cutoff freq: fh"="fh Top", "sampling freq: fs"=w1304, "X"=w1301) -> ("Filtered X"=w1330:dbl[])  [unwired: 1 in, 1 out]
    n875 = call-poly <vilib>:"Butterworth Filter.vi"("init/cont (init:F)"=TRUE, "order"=3, "filter type"="top filter", "low cutoff freq: fl"="fl Top", "high cutoff freq: fh"="fh Top", "sampling freq: fs"=w1304, "X"=w1263) -> ("Filtered X"=w1255:dbl[])  [unwired: 1 in, 1 out]
    n876 = call-poly <vilib>:"Butterworth Filter.vi"("init/cont (init:F)"=TRUE, "order"=3, "filter type"="bottom filter", "low cutoff freq: fl"="fl Bottom", "high cutoff freq: fh"="fh Bottom", "sampling freq: fs"=w1304, "X"=w1300) -> ("Filtered X"=w1331:dbl[])  [unwired: 1 in, 1 out]
    n877 = call-poly <vilib>:"Butterworth Filter.vi"("init/cont (init:F)"=TRUE, "order"=3, "filter type"="bottom filter", "low cutoff freq: fl"="fl Bottom", "high cutoff freq: fh"="fh Bottom", "sampling freq: fs"=w1304, "X"=w1262) -> ("Filtered X"=w1254:dbl[])  [unwired: 1 in, 1 out]
    n878 = Build Array(w1299, w1332, w1330, w1331, w1257, w1256, w1255, w1254) -> (→"8 Ch Heart":dbl[][])
  }
  n879 = while {
    tunnel: w41 -> [w1386]
    tunnel: w32 -> [w1385]
    tunnel: w2 -> [w1381]
    stop <- FALSE stop-if-true
    n880 = Wait (ms)(milliseconds to wait=u32 100) -> ()  [unwired: 1 out]
    n881 = Get Queue Status(queue=w1386) -> (queue out=w1388:refnum<queue>, # elements in queue=w1389:i32)  [unwired: 2 in, 6 out]
    "# NCS Buffer" <- w1389
    n882 = Get Queue Status(queue=w1381) -> (queue out=w1382:refnum<queue>, # elements in queue=w1380:i32)  [unwired: 2 in, 6 out]
    n883 = local read "Save"() -> (w1383:bool)
    n884 = case shown="True" w1383 {
      tunnel: w1389 -> [_ w1461]
      tunnel: w1388 -> [_ w1462]
      tunnel: w1385 -> [_ w1460]
      tunnel: w1382 -> [_ w1399]
      tunnel: w1380 -> [_ w1394]
      frame False {
      }
      frame True {
        # "Once Saved: Stop saving"
        # "Getting channels from Buffer Queue"
        n885 = Multiply(x=w1461, y=w1460) -> (x*y=w1415:dbl)
        n886 = for {
          N: w1461 -> [_]
          tunnel: [w1654] -> w1431 mode=indexing
          tunnel: [w1650] -> w1430 mode=indexing
          tunnel: [w1649] -> w1428 mode=indexing
          tunnel: [w1648] -> w1426 mode=indexing
          shift-right: [w1646] -> _
          shift-left: w1462 -> [w1656]
          tunnel: [w1641] -> w1420 mode=indexing
          tunnel: [w1640] -> w1419 mode=indexing
          tunnel: [w1639] -> w1418 mode=indexing
          tunnel: [w1638] -> w1417 mode=indexing
          tunnel: [w1629] -> w1416 mode=indexing
          tunnel: [w1627] -> w1414 mode=indexing
          tunnel: [w1626] -> w1413 mode=indexing
          tunnel: [w1625] -> w1412 mode=indexing
          tunnel: [w1624] -> w1411 mode=indexing
          tunnel: [w1623] -> w1410 mode=indexing
          tunnel: [w1622] -> w1409 mode=indexing
          tunnel: [w1621] -> w1408 mode=indexing
          i -> [w1647]
          n887 = Dequeue Element(queue=w1656) -> (queue out=w1646:refnum<queue>, element=w1628:dbl[][])  [unwired: 2 in, 2 out]
          n888 = Index Array(array=w1628, index (row)=13) -> (element=w1623:dbl[])  [unwired: 1 in]
          n889 = Index Array(array=w1628, index (row)=14) -> (element=w1622:dbl[])  [unwired: 1 in]
          n890 = Index Array(array=w1628, index (row)=15) -> (element=w1621:dbl[])  [unwired: 1 in]
          n891 = Index Array(array=w1628, index (row)=9) -> (element=w1627:dbl[])  [unwired: 1 in]
          n892 = Index Array(array=w1628, index (row)=10) -> (element=w1626:dbl[])  [unwired: 1 in]
          n893 = Index Array(array=w1628, index (row)=11) -> (element=w1625:dbl[])  [unwired: 1 in]
          n894 = Index Array(array=w1628, index (row)=12) -> (element=w1624:dbl[])  [unwired: 1 in]
          n895 = Index Array(array=w1628, index (row)=5) -> (element=w1640:dbl[])  [unwired: 1 in]
          n896 = Index Array(array=w1628, index (row)=6) -> (element=w1639:dbl[])  [unwired: 1 in]
          n897 = Index Array(array=w1628, index (row)=7) -> (element=w1638:dbl[])  [unwired: 1 in]
          n898 = Index Array(array=w1628, index (row)=8) -> (element=w1629:dbl[])  [unwired: 1 in]
          n899 = Index Array(array=w1628, index (row)=4) -> (element=w1641:dbl[])  [unwired: 1 in]
          n900 = Index Array(array=w1628, index (row)=1) -> (element=w1650:dbl[])  [unwired: 1 in]
          n901 = Index Array(array=w1628, index (row)=2) -> (element=w1649:dbl[])  [unwired: 1 in]
          n902 = Index Array(array=w1628, index (row)=3) -> (element=w1648:dbl[])  [unwired: 1 in]
          n903 = Index Array(array=w1628, index (row)=0) -> (element=w1654:dbl[])  [unwired: 1 in]
          "NCS Save Loops" <- w1647
        }
        n904 = for {
          N: w1394 -> [_]
          tunnel: [w1471] -> w1396 mode=concatenating
          tunnel: [w1468] -> w1397 mode=concatenating
          tunnel: [w1467] -> w1398 mode=concatenating
          tunnel: w1399 -> [w1464]
          tunnel: [w1463] -> w1395 mode=concatenating
          n905 = Dequeue Element(queue=w1464) -> (element=w1465:dbl[][])  [unwired: 2 in, 3 out]
          n906 = Index Array(array=w1465, index (row)=0) -> (element=w1467:dbl[])  [unwired: 1 in]
          n907 = Index Array(array=w1465, index (row)=1) -> (element=w1468:dbl[])  [unwired: 1 in]
          n908 = Index Array(array=w1465, index (row)=2) -> (element=w1471:dbl[])  [unwired: 1 in]
          n909 = Index Array(array=w1465, index (row)=3) -> (element=w1463:dbl[])  [unwired: 1 in]
        }
        n910 = local read "Current Routine"() -> (w1457:string)
        n911 = local read "Case #"() -> (w1392:string)
        n912 = Format Date/Time String(time format string (%c)="%m%d_%H%M%S") -> (date/time string=w1458:string)  [unwired: 2 in]
        n913 = Concatenate Strings("Case", w1392, "_", w1458, w1457) -> (w1390:string)
        n914 = flat-sequence {
          tunnel: w1433 -> [w1555]
          tunnel: w1434 -> [w1556]
          tunnel: w1435 -> [w1557]
          tunnel: w1436 -> [w1558]
          tunnel: w1437 -> [w1560]
          tunnel: w1438 -> [w1559]
          tunnel: w1439 -> [w1561]
          tunnel: w1440 -> [w1562]
          tunnel: w1441 -> [w1563]
          tunnel: w1442 -> [w1564]
          tunnel: w1443 -> [w1565]
          tunnel: w1444 -> [w1566]
          tunnel: w1445 -> [w1567]
          tunnel: w1446 -> [w1568]
          tunnel: "Abd (cm)" -> [w1590]
          tunnel: "Comments" -> [w1585]
          tunnel: "Weight (lbs)" -> [w1586]
          tunnel: "Thorax (cm)" -> [w1588]
          tunnel: "Height (cm)" -> [w1593]
          tunnel: "Age (yrs)" -> [w1595]
          tunnel: "Sex" -> [w1597]
          tunnel: "Case #" -> [w1598]
          tunnel: path "C:/Users/Edwin Kan Group/Documents/Zijing/dyspnea study/data/10_12" ("base path") -> [w1619]
          tunnel: w1390 -> [w1618]
          tunnel: w1432 -> [w1554]
          tunnel: w1425 -> [w1541]
          tunnel: w1427 -> [w1544]
          tunnel: w1429 -> [w1549]
          tunnel: w1424 -> [w1540]
          tunnel: w1423 -> [w1537]
          tunnel: w1422 -> [w1532]
          tunnel: w1421 -> [w1531]
          tunnel: w1407 -> [w1526]
          tunnel: w1406 -> [w1523]
          tunnel: w1405 -> [w1520]
          tunnel: w1404 -> [w1517]
          tunnel: w1403 -> [w1516]
          tunnel: w1402 -> [w1509]
          tunnel: w1401 -> [w1508]
          tunnel: w1400 -> [w1507]
          tunnel: w1398 -> [w1480]
          tunnel: w1397 -> [w1478]
          tunnel: w1396 -> [w1476]
          tunnel: w1395 -> [w1474]
          frame #0 {
            n915 = Build Path(base path=w1619, name or relative path=w1618) -> (appended path=w1601:path)
            n916 = TDMS Open(6:FALSE ("disable buffering (T)"), 10:T9."open or create" ("operation"), 11:w1601) -> (0:w1616:errorcluster, 3:w1617:refnum<k34>)  [unwired: 4 in]
            n917 = TDMS Set Properties(5:w1598, 7:"Case Number", 8:w1616, 11:w1617) -> (0:w1615:errorcluster, 3:w1614:refnum<k34>)  [unwired: 2 in, 2 out]
            n918 = TDMS Set Properties(5:w1597, 7:"Sex", 8:w1615, 11:w1614) -> (0:w1613:errorcluster, 3:w1612:refnum<k34>)  [unwired: 2 in, 2 out]
            n919 = TDMS Set Properties(5:w1595, 7:"Age (years)", 8:w1613, 11:w1612) -> (0:w1611:errorcluster, 3:w1610:refnum<k34>)  [unwired: 2 in, 2 out]
            n920 = TDMS Set Properties(5:w1593, 7:"Height (cm)", 8:w1611, 11:w1610) -> (0:w1608:errorcluster, 3:w1607:refnum<k34>)  [unwired: 2 in, 2 out]
            n921 = TDMS Set Properties(5:w1590, 7:"AbdCircumference (cm)", 8:w1608, 11:w1607) -> (0:w1606:errorcluster, 3:w1605:refnum<k34>)  [unwired: 2 in, 2 out]
            n922 = TDMS Set Properties(5:w1588, 7:"Thorax Circumference (cm)", 8:w1606, 11:w1605) -> (0:w1603:errorcluster, 3:w1604:refnum<k34>)  [unwired: 2 in, 2 out]
            n923 = TDMS Set Properties(5:w1586, 7:"Weight (lbs)", 8:w1603, 11:w1604) -> (0:w1587:errorcluster, 3:w1609:refnum<k34>)  [unwired: 2 in, 2 out]
            n924 = TDMS Set Properties(5:w1585, 7:"Comments", 8:w1587, 11:w1609) -> (0:w1569:errorcluster, 3:w1570:refnum<k34>)  [unwired: 2 in, 2 out]
            n925 = TDMS Set Properties(5:w1567, 7:w1568, 8:w1569, 11:w1570) -> (0:w1582:errorcluster, 3:w1581:refnum<k34>)  [unwired: 2 in, 2 out]
            n926 = TDMS Set Properties(5:w1565, 7:w1566, 8:w1582, 11:w1581) -> (0:w1580:errorcluster, 3:w1579:refnum<k34>)  [unwired: 2 in, 2 out]
            n927 = TDMS Set Properties(5:w1563, 7:w1564, 8:w1580, 11:w1579) -> (0:w1577:errorcluster, 3:w1576:refnum<k34>)  [unwired: 2 in, 2 out]
            n928 = TDMS Set Properties(5:w1561, 7:w1562, 8:w1577, 11:w1576) -> (0:w1575:errorcluster, 3:w1574:refnum<k34>)  [unwired: 2 in, 2 out]
            n929 = TDMS Set Properties(5:w1559, 7:w1560, 8:w1575, 11:w1574) -> (0:w1572:errorcluster, 3:w1573:refnum<k34>)  [unwired: 2 in, 2 out]
            n930 = TDMS Set Properties(5:w1557, 7:w1558, 8:w1572, 11:w1573) -> (0:w1571:errorcluster, 3:w1578:refnum<k34>)  [unwired: 2 in, 2 out]
            n931 = TDMS Set Properties(5:w1555, 7:w1556, 8:w1571, 11:w1578) -> (0:w1552:errorcluster, 3:w1553:refnum<k34>)  [unwired: 2 in, 2 out]
            n932 = TDMS Write(0:w1553, 7:"Tx1Rx1", 9:w1554, 11:w1552) -> (4:w1550:refnum<k34>, 15:w1551:errorcluster)  [unwired: 2 in, 2 out]
            n933 = TDMS Write(0:w1550, 7:"Tx2Rx1", 9:w1549, 11:w1551) -> (4:w1545:refnum<k34>, 15:w1546:errorcluster)  [unwired: 2 in, 2 out]
            n934 = TDMS Write(0:w1545, 7:"Tx3Rx1", 9:w1544, 11:w1546) -> (4:w1542:refnum<k34>, 15:w1543:errorcluster)  [unwired: 2 in, 2 out]
            n935 = TDMS Write(0:w1542, 7:"Tx4Rx1", 9:w1541, 11:w1543) -> (4:w1538:refnum<k34>, 15:w1539:errorcluster)  [unwired: 2 in, 2 out]
            n936 = TDMS Write(0:w1538, 7:"Tx1Rx2", 9:w1540, 11:w1539) -> (4:w1535:refnum<k34>, 15:w1536:errorcluster)  [unwired: 2 in, 2 out]
            n937 = TDMS Write(0:w1535, 7:"Tx2Rx2", 9:w1537, 11:w1536) -> (4:w1533:refnum<k34>, 15:w1534:errorcluster)  [unwired: 2 in, 2 out]
            n938 = TDMS Write(0:w1533, 7:"Tx3Rx2", 9:w1532, 11:w1534) -> (4:w1529:refnum<k34>, 15:w1530:errorcluster)  [unwired: 2 in, 2 out]
            n939 = TDMS Write(0:w1529, 7:"Tx4Rx2", 9:w1531, 11:w1530) -> (4:w1527:refnum<k34>, 15:w1528:errorcluster)  [unwired: 2 in, 2 out]
            n940 = TDMS Write(0:w1527, 7:"Tx1Rx3", 9:w1526, 11:w1528) -> (4:w1524:refnum<k34>, 15:w1525:errorcluster)  [unwired: 2 in, 2 out]
            n941 = TDMS Write(0:w1524, 7:"Tx2Rx3", 9:w1523, 11:w1525) -> (4:w1522:refnum<k34>, 15:w1519:errorcluster)  [unwired: 2 in, 2 out]
            n942 = TDMS Write(0:w1522, 7:"Tx3Rx3", 9:w1520, 11:w1519) -> (4:w1521:refnum<k34>, 15:w1518:errorcluster)  [unwired: 2 in, 2 out]
            n943 = TDMS Write(0:w1521, 7:"Tx4Rx3", 9:w1517, 11:w1518) -> (4:w1514:refnum<k34>, 15:w1515:errorcluster)  [unwired: 2 in, 2 out]
            n944 = TDMS Write(0:w1514, 7:"Tx1Rx4", 9:w1516, 11:w1515) -> (4:w1513:refnum<k34>, 15:w1512:errorcluster)  [unwired: 2 in, 2 out]
            n945 = TDMS Write(0:w1513, 7:"Tx2Rx4", 9:w1509, 11:w1512) -> (4:w1510:refnum<k34>, 15:w1511:errorcluster)  [unwired: 2 in, 2 out]
            n946 = TDMS Write(0:w1510, 7:"Tx3Rx4", 9:w1508, 11:w1511) -> (4:w1505:refnum<k34>, 15:w1506:errorcluster)  [unwired: 2 in, 2 out]
            n947 = TDMS Write(0:w1505, 7:"Tx4Rx4", 9:w1507, 11:w1506) -> (4:w1490:refnum<k34>, 15:w1485:errorcluster)  [unwired: 2 in, 2 out]
            n948 = TDMS Write(0:w1490, 7:"BIOPAC_CH1", 9:w1480, 11:w1485) -> (4:w1489:refnum<k34>, 15:w1484:errorcluster)  [unwired: 2 in, 2 out]
            n949 = TDMS Write(0:w1489, 7:"BIOPAC_CH2", 9:w1478, 11:w1484) -> (4:w1488:refnum<k34>, 15:w1483:errorcluster)  [unwired: 2 in, 2 out]
            n950 = TDMS Write(0:w1488, 7:"BIOPAC_CH3", 9:w1476, 11:w1483) -> (4:w1487:refnum<k34>, 15:w1482:errorcluster)  [unwired: 2 in, 2 out]
            n951 = TDMS Write(0:w1487, 7:"BIOPAC_CH4", 9:w1474, 11:w1482) -> (4:w1486:refnum<k34>, 15:w1481:errorcluster)  [unwired: 2 in, 2 out]
            n952 = TDMS Close(8:w1481, 11:w1486) -> ()  [unwired: 2 out]
          }
          frame #1 {
            n953 = local write "Save"(FALSE) -> ()
          }
        }
        n954 = local read "Start Time"() -> (w1449:T2)
        n955 = property on="fractional second" class="DigNum (strict)"() -> ("Label.Text"=w1446:string)  [unwired: 2 in, 2 out]
        n956 = property on="second" class="DigNum (strict)"() -> ("Label.Text"=w1444:string)  [unwired: 2 in, 2 out]
        n957 = Unbundle By Name(w1449) -> ("fractional second"=w1445:dbl, "second"=w1443:i32, "minute"=w1441:i32, "hour"=w1439:i32, "day of month"=w1438:i32, "month"=w1435:i32, "year"=w1433:i32)
        n958 = property on="minute" class="DigNum (strict)"() -> ("Label.Text"=w1442:string)  [unwired: 2 in, 2 out]
        n959 = property on="hour" class="DigNum (strict)"() -> ("Label.Text"=w1440:string)  [unwired: 2 in, 2 out]
        n960 = property on="month" class="DigNum (strict)"() -> ("Label.Text"=w1436:string)  [unwired: 2 in, 2 out]
        n961 = property on="day of month" class="DigNum (strict)"() -> ("Label.Text"=w1437:string)  [unwired: 2 in, 2 out]
        n962 = property on="year" class="DigNum (strict)"() -> ("Label.Text"=w1434:string)  [unwired: 2 in, 2 out]
        n963 = Reshape Array(w1431, w1415) -> (w1432:dbl[])
        n964 = Reshape Array(w1430, w1415) -> (w1429:dbl[])
        n965 = Reshape Array(w1428, w1415) -> (w1427:dbl[])
        n966 = Reshape Array(w1426, w1415) -> (w1425:dbl[])
        n967 = Reshape Array(w1420, w1415) -> (w1424:dbl[])
        n968 = Reshape Array(w1419, w1415) -> (w1423:dbl[])
        n969 = Reshape Array(w1418, w1415) -> (w1422:dbl[])
        n970 = Reshape Array(w1417, w1415) -> (w1421:dbl[])
        n971 = Reshape Array(w1416, w1415) -> (w1407:dbl[])
        n972 = Reshape Array(w1414, w1415) -> (w1406:dbl[])
        n973 = Reshape Array(w1413, w1415) -> (w1405:dbl[])
        n974 = Reshape Array(w1412, w1415) -> (w1404:dbl[])
        n975 = Reshape Array(w1411, w1415) -> (w1403:dbl[])
        n976 = Reshape Array(w1410, w1415) -> (w1402:dbl[])
        n977 = Reshape Array(w1409, w1415) -> (w1401:dbl[])
        n978 = Reshape Array(w1408, w1415) -> (w1400:dbl[])
      }
    }
  }
  n979 = while {
    stop <- FALSE stop-if-true
    # "Viewing NCS"
    n980 = local read "8 Ch Heart"() -> (w1664:dbl[][])
    n981 = Index Array(array=w1664, index (row)=6 ("index")) -> (element=→"Tx4Rx4":dbl[])  [unwired: 1 in]
    n982 = Index Array(array=w1664, index (row)=7 ("index")) -> (element=→"Tx3Rx4":dbl[])  [unwired: 1 in]
    n983 = Index Array(array=w1664, index (row)=3 ("index")) -> (element=→"Tx1Rx2":dbl[])  [unwired: 1 in]
    n984 = Index Array(array=w1664, index (row)=2 ("index")) -> (element=→"Tx2Rx2":dbl[])  [unwired: 1 in]
    n985 = Index Array(array=w1664, index (row)=0 ("index")) -> (element=→"Tx1Rx1":dbl[])  [unwired: 1 in]
    n986 = Index Array(array=w1664, index (row)=5 ("index")) -> (element=→"Tx4Rx3":dbl[])  [unwired: 1 in]
    n987 = Index Array(array=w1664, index (row)=4 ("index")) -> (element=→"Tx3Rx3":dbl[])  [unwired: 1 in]
    n988 = Index Array(array=w1664, index (row)=1 ("index")) -> (element=→"Tx2Rx1":dbl[])  [unwired: 1 in]
    n989 = Wait (ms)(milliseconds to wait=u32 30) -> ()  [unwired: 1 out]
  }
  "error out 1" <- w169
  "error out 2" <- w103
  "DownSamplingRatio" <- "DownSamplingRatio1"
  "ACQ ms" <- 100.0
  "Connecting" <- w1
  "Stopping" <- w1
  "Disconnecting" <- w1
  "Boolean" <- TRUE
  "Disconnected" <- w1
  "Connected" <- w1
  "Receive Success" <- w1
  "Receiving" <- w1
  "Acq Started" <- w1
